vi "CRYGraph Property Window XY.vi"(9 "TabName":string, 10 "Graph VI Ref":refnum<vi>) -> ()   [LabVIEW 2013]
uses:
  <vilib>/Utility/miscctls.llb/LVRowAndColumnTypeDef.ctl
panel:
  in  "Plot PropertyCtrl Ref":refnum<vi>
  in  "Plot Property":string
  in  "SetFormat":bool
  in  "No Data":bool
  out "CursorLineStyle":string
  out "CursorLineWidth":string
  out "CursorPointStyle":string
  out "CursorStyle":string
  out "Scale Style":u8=5
  out "Interpolation":string
  out "PointStyle":string
  out "LineWidth":string
  out "LineStyle":string
  in  "Property Tab":T1(tab)
  in  "Background Color":u32(colorbox)
  in  "Title Name":string
  in  "FormatAxis":u16(ring) items=["X-Axis", "Y-Axis"]
  in  "Notation":i32(listbox)
  in  "PrecisionType":u16(ring) items=["Digitals of precision", "Significant digits"]
  in  "PrecisionDigits":u16
  in  "Hide trailing zeros":bool
  in  "Exponent in multiples of 3":bool
  in  "Use minimum field width":bool
  in  "Field Width":u16
  in  "PadType":u16(ring) items=["Pad with spaces on left", "Pad with spaces on right", "Pad with zeros on left"]
  in  "Ignore timestamp information":bool
  in  "TimeFormat":u16(ring) items=["Custom time format", "System time format", "Time unused"]
  in  "Digits":u16
  in  "DateFormat":u16(ring) items=["Custom date format", "System date format", "Date unused"]
  in  "YMD":u16(slide)
  in  "YearShow":u16(slide)
  in  "AMFM":u16(slide)=1
  in  "HMS":u16(slide)=1
  in  "Point/Fill":u32(colorbox)
  in  "Fill to":i16(ring) items=["none"=-1, "zero"=-2, "-Infinity"=-3, "+Infinity"=-4]
  in  "Items":u16(ring)
  out "Colors":bool
  in  "Line":u32(colorbox)
  in  "LineStyle4":bool
  in  "LineStyle3":bool
  in  "LineStyle2":bool
  in  "LineStyle0":bool
  in  "LineStyle1":bool
  in  "LineWidth5":bool
  in  "LineWidth1":bool
  in  "LineWidth4":bool
  in  "LineWidth3":bool
  in  "LineWidth2":bool
  in  "LineWidth0":bool
  in  "PointStyle16":bool
  in  "PointStyle15":bool
  in  "PointStyle14":bool
  in  "PointStyle13":bool
  in  "PointStyle12":bool
  in  "PointStyle11":bool
  in  "PointStyle10":bool
  in  "PointStyle9":bool
  in  "PointStyle8":bool
  in  "PointStyle7":bool
  in  "PointStyle6":bool
  in  "PointStyle5":bool
  in  "PointStyle4":bool
  in  "PointStyle3":bool
  in  "PointStyle2":bool
  in  "PointStyle1":bool
  in  "PointStyle0":bool
  in  "Interpolation4":bool
  in  "Interpolation5":bool
  in  "Interpolation3":bool
  in  "Interpolation2":bool
  in  "Interpolation1":bool
  in  "Interpolation0":bool
  in  "Show Plot":bool
  in  "GridStyle":u16(ring)=4
  out "Grid Colors":bool
  in  "Minor grid":u32(colorbox)
  in  "Major grid":u32(colorbox)
  in  "Marker text":u32(colorbox)
  in  "Minor tick":u32(colorbox)
  in  "Log":bool
  in  "Show scale":bool
  in  "Show scale label":bool
  in  "Maximum":dbl
  in  "Minimum":dbl
  in  "Autoscale":bool
  in  "Axis Name":string caption="Name"
  in  "Axis":u16(ring)
  in  "Major tick":u32(colorbox)
  out "Scale Style and Colors":bool
  in  "Cursor Tab":enum32{"Page 1"}(tab)
  in  "CursorPointStyle16":bool
  in  "CursorPointStyle15":bool
  in  "CursorPointStyle14":bool
  in  "CursorPointStyle13":bool
  in  "CursorPointStyle12":bool
  in  "CursorPointStyle11":bool
  in  "CursorPointStyle10":bool
  in  "CursorPointStyle9":bool
  in  "CursorPointStyle8":bool
  in  "CursorPointStyle7":bool
  in  "CursorPointStyle6":bool
  in  "CursorPointStyle5":bool
  in  "CursorPointStyle4":bool
  in  "CursorPointStyle3":bool
  in  "CursorPointStyle2":bool
  in  "CursorPointStyle1":bool
  in  "CursorPointStyle0":bool
  in  "CursorLineWidth5":bool
  in  "CursorLineWidth1":bool
  in  "CursorLineWidth4":bool
  in  "CursorLineWidth3":bool
  in  "CursorLineWidth2":bool
  in  "CursorLineWidth0":bool
  in  "CursorLineStyle4":bool
  in  "CursorLineStyle3":bool
  in  "CursorLineStyle2":bool
  in  "CursorLineStyle0":bool
  in  "CursorLineStyle1":bool
  in  "Cursor Items":u16(ring)
  in  "CursorStyle8":bool
  in  "CursorStyle4":bool
  in  "CursorStyle5":bool
  in  "CursorStyle7":bool
  in  "CursorStyle6":bool
  in  "CursorStyle3":bool
  in  "CursorStyle2":bool
  in  "CursorStyle1":bool
  in  "CursorStyle0":bool
  in  "Cursor color":u32(colorbox)
  in  "Linked to plot:":u16(ring)
  in  "Link Cursors":bool
  in  "Show Cursors":bool
  in  "OK":bool
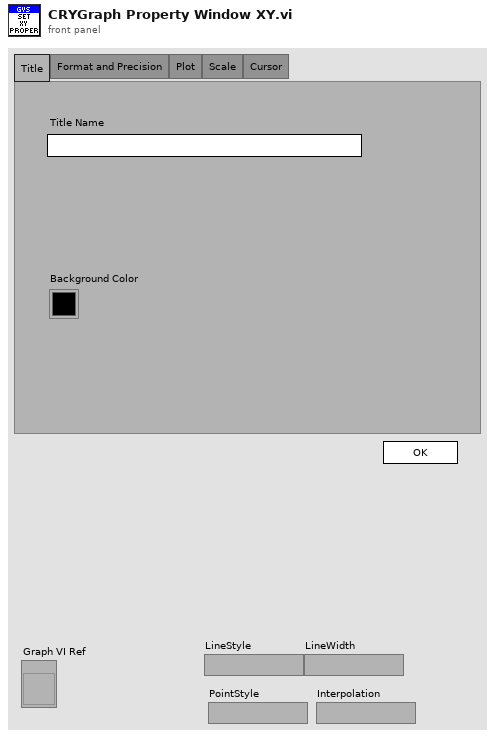
[diagram p1: front panel]
types:
  T1 = enum32{"Title", "Format and Precision", "Plot", "Scale", "Cursor"}
  T2 = enum32{"Page Enabled", "Page Disabled", "Page Disabled & Grayed"}
  T3 = enum8{"Enabled", "Disabled", "Disabled and Grayed Out"}
  T4 = typedef "LVRowAndColumnTypeDef.ctl" = cluster{"Row":i32, "Column":i32}
  T5 = typedef "CRYData Cluster.ctl" = cluster{"Name":string, "Curve":cluster{"x":dbl, "y":dbl, "z":dbl}[], "X data":u16, "Y data":u16, "Z data":u16, "X axis":u16, "Y axis":u16, "Z axis":u16, "X unit":string, "Y unit":string, "Z unit":string, "X dB ref":dbl, "Y dB ref":dbl, "Z dB ref":dbl, "single val":bool, "protected":bool, "display X":bool, "display Y":bool, "display Z":bool, "Test Info":string, "Step No.":i32, "Plot Settings":cluster{"Color":u32, "Interpolation":u8, "Point Style":u8, "Line Style":u8, "Point Color":u32, "Line Width":u8, "Bar Plot Style":u8, "Fill To":i16}, "AutoProtect":bool}
  T6 = cluster{"Notation":i32, "PrecisionType":u16, "PrecisionDigits":u16, "Hide trailing zeros":bool, "Exponent in multiples of 3":bool, "Field Width":u16, "PadType":u16, "Use minimum field width":bool, "TimeFormat":u16, "AMFM":u16, "HMS":u16, "Digits":u16, "DateFormat":u16, "YMD":u16, "YearShow":u16}
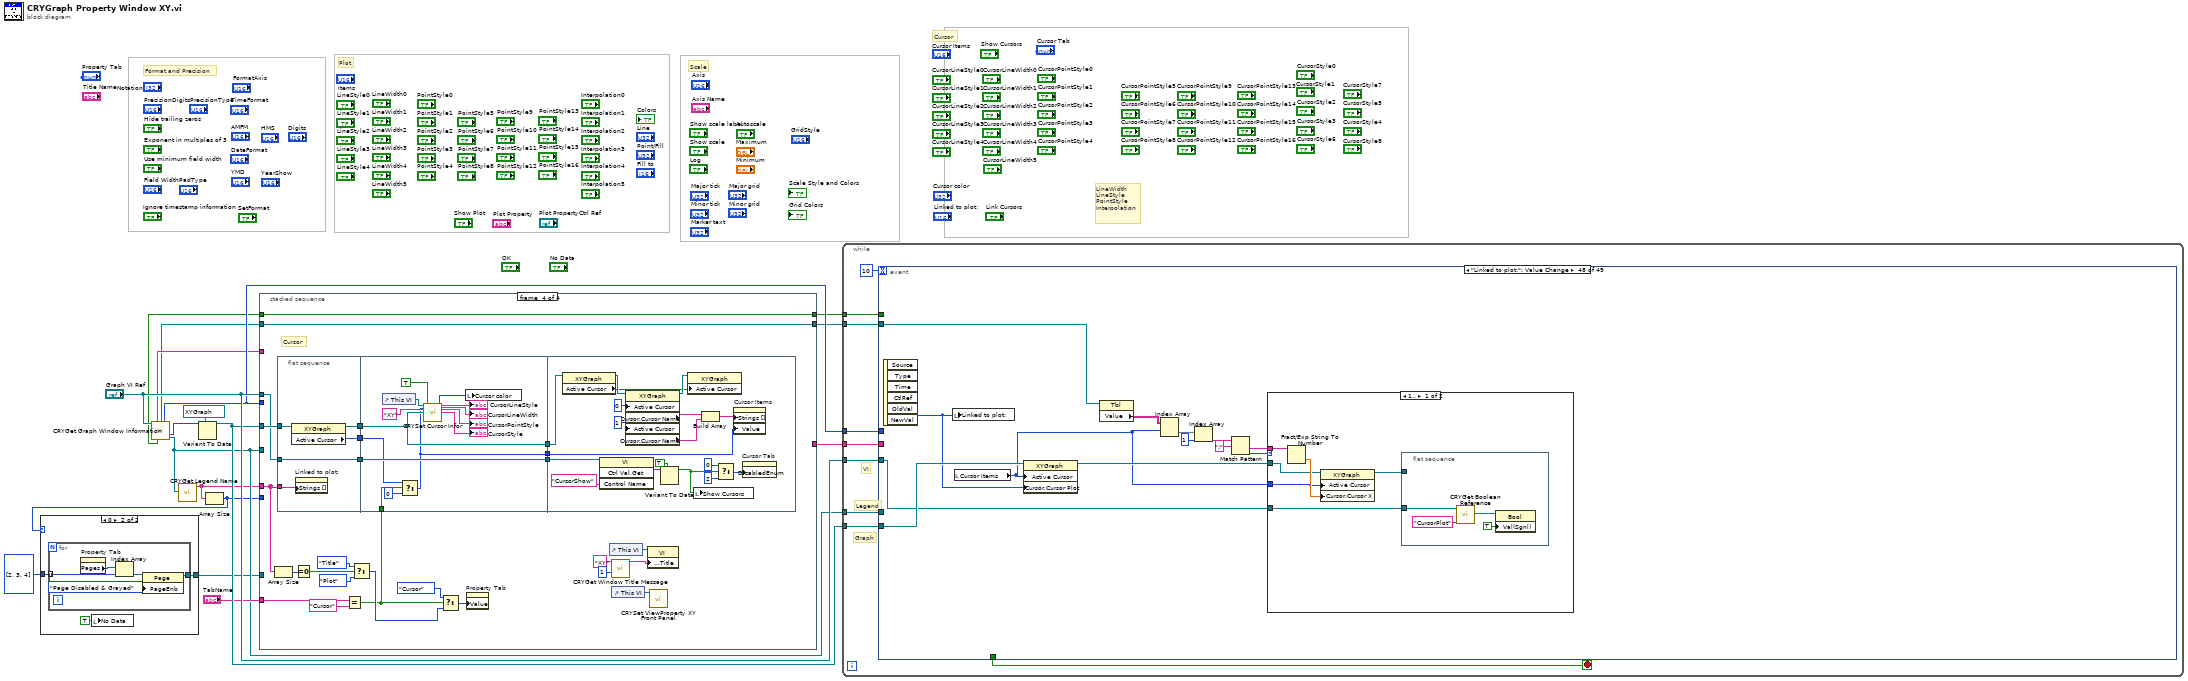
[diagram p0: block diagram]
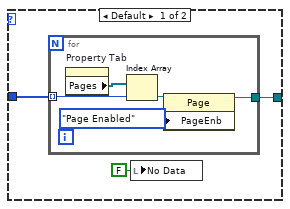
[diagram p2: hidden frame]
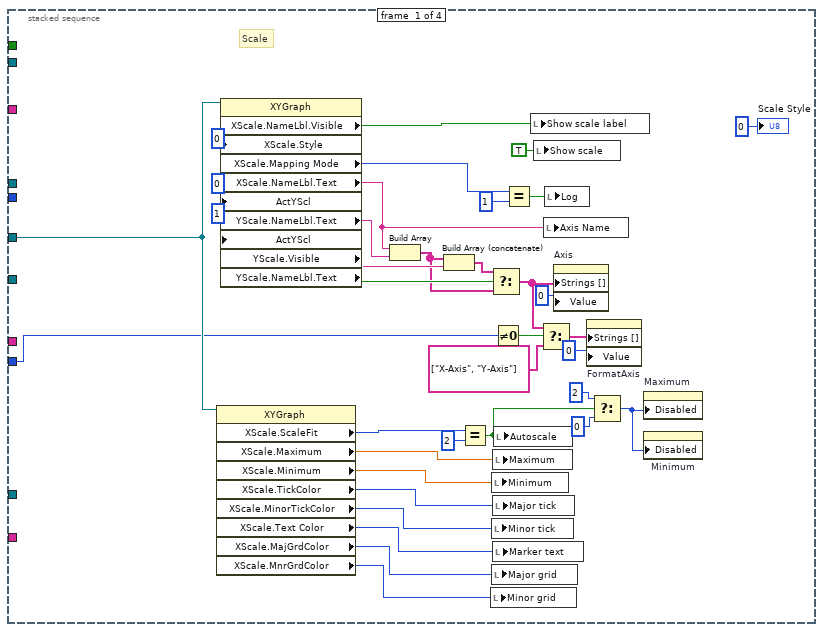
[diagram p3: hidden frame]
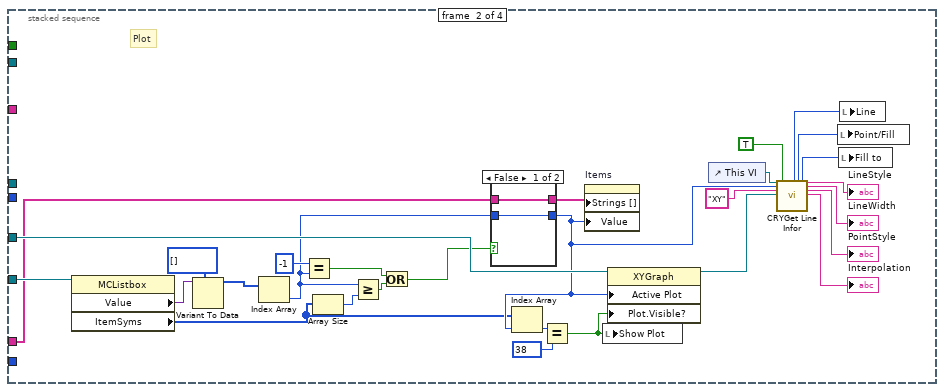
[diagram p4: hidden frame]
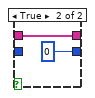
[diagram p5: hidden frame]
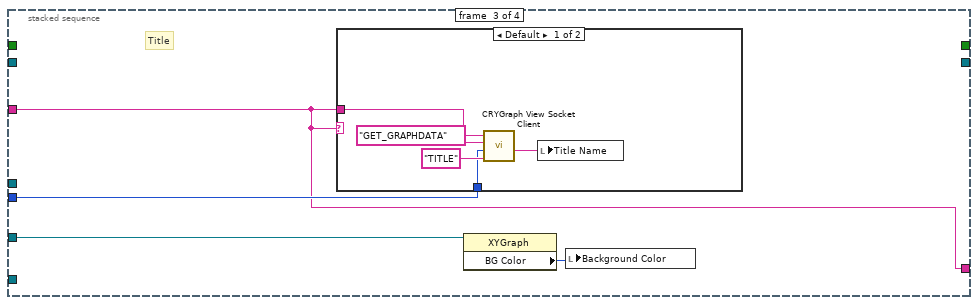
[diagram p6: hidden frame]
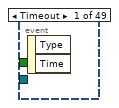
[diagram p8: hidden frame]
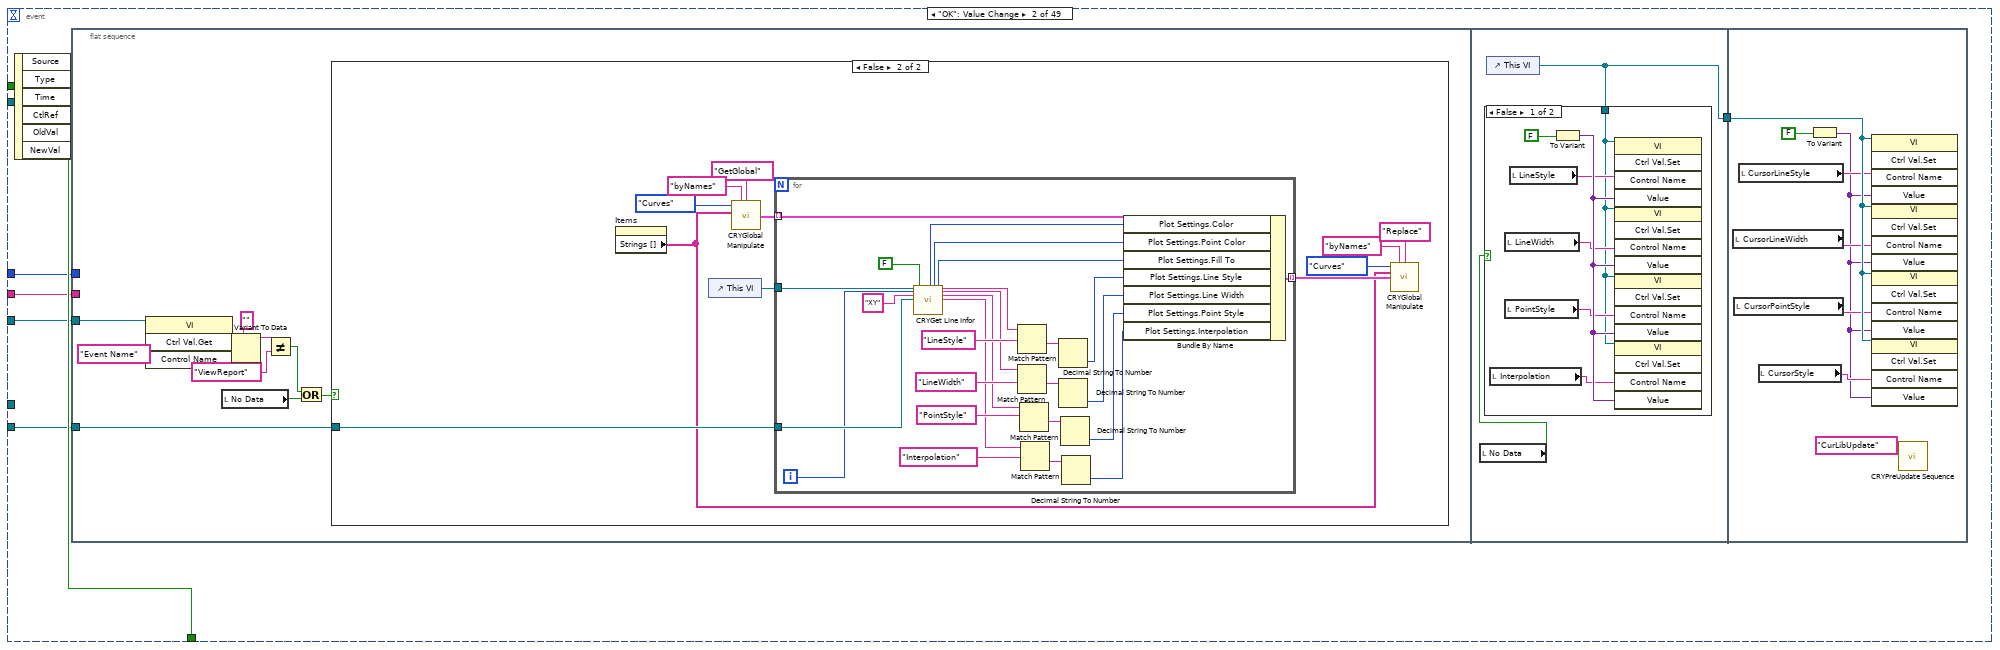
[diagram p9: hidden frame]
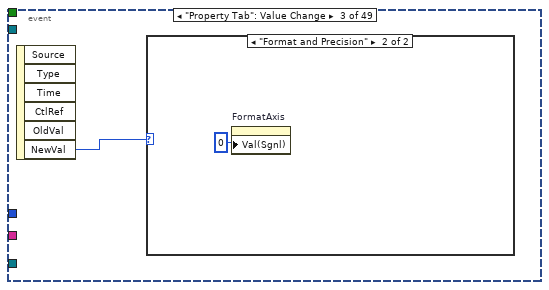
[diagram p12: hidden frame]
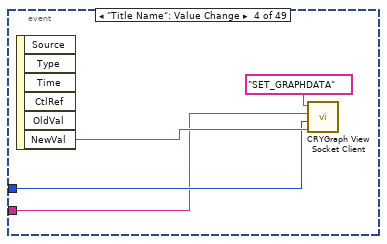
[diagram p14: hidden frame]
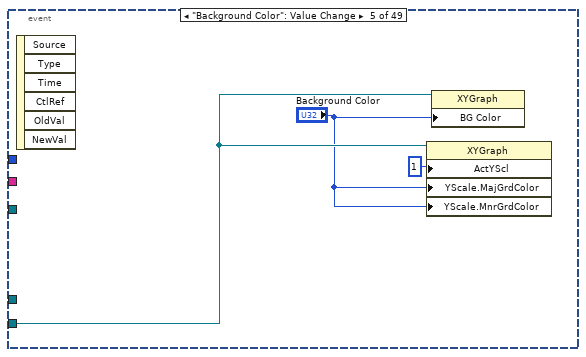
[diagram p15: hidden frame]
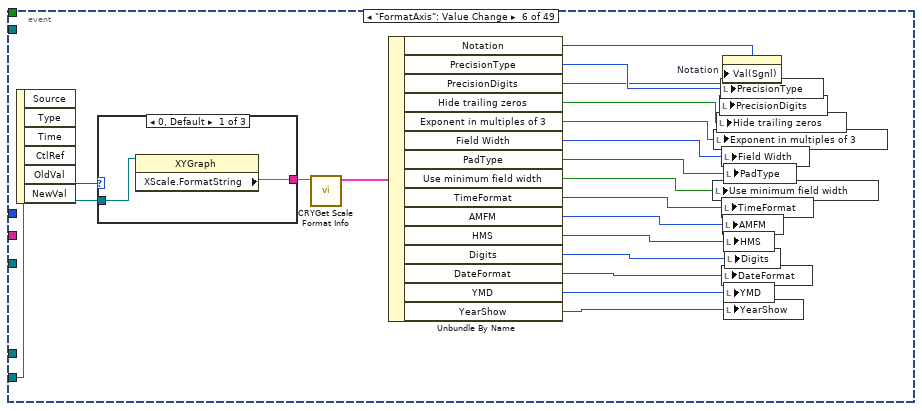
[diagram p16: hidden frame]
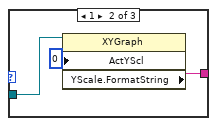
[diagram p17: hidden frame]
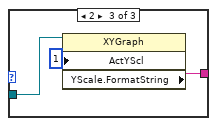
[diagram p18: hidden frame]
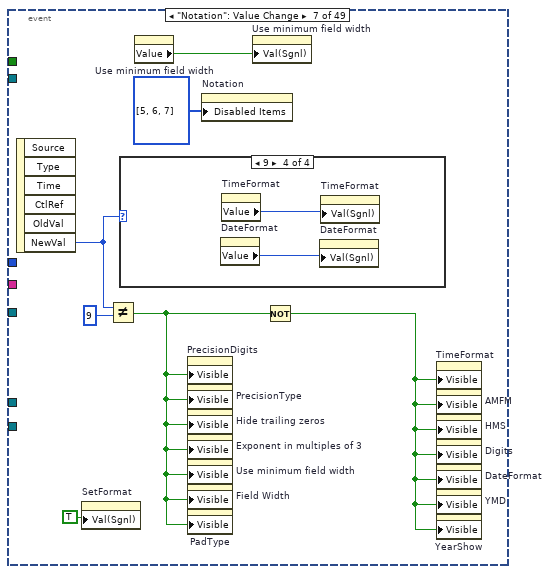
[diagram p19: hidden frame]
diagram:
  # "LineWidth\nLineStyle\nPointStyle\nInterpolation"
  # "Format and Precision"
  # "Cursor"
  # "Scale"
  # "Plot"
  n1 = call "CRYGet Graph Window Information.vi"("pGraph VI In"="Graph VI Ref") -> ("Queue Name Out"=w14:string, "Cursor Ref Out"=w4:refnum<vi>, "Graph Number Out"=w15:i32, "Graph Control Ref Out"=w6:variant, "CursorShow Out"=w2:bool, "Legend Ref Out"=w11:refnum<vi>)  [unwired: 2 in, 7 out]
  n2 = call "CRYGet Legend Name.vi"("MCListbox Refnum"=w11) -> ("Names Out"=w10:string[])  [unwired: 1 in, 9 out]
  n3 = Variant To Data(type=refnum<vi> refnum ("XY Graph"), Variant=w6) -> (data=w16:refnum<vi>)  [unwired: 1 in, 1 out]
  n4 = Array Size(array=w10) -> (size(s)=w9:i32)
  n5 = case shown="0" w9 {
    tunnel: i32[] [2, 3, 4] -> [w19 w27]
    tunnel: [w18 w26] -> w8
    frame Default {
      n6 = for {
        tunnel: w19 -> [w23] mode=indexing
        tunnel: [w21] -> w18
        n7 = property on="Property Tab" class="TabCtl (strict)"() -> ("Pages"=w22:refnum<vi>[])  [unwired: 2 in, 2 out]
        n8 = Index Array(array=w22, index=w23) -> (element=w24:refnum<vi>)
        n9 = property class="Page"(reference=w24, "PageEnb"=T2."Page Enabled" ("Page Enabled State")) -> (reference out=w21:refnum<vi>)  [unwired: 1 in, 1 out]
      }
      n10 = local write "No Data"(FALSE ("No Data")) -> ()
    }
    frame 0 {
      n11 = for {
        tunnel: w27 -> [w30] mode=indexing
        tunnel: [w29] -> w26
        n12 = property on="Property Tab" class="TabCtl (strict)"() -> ("Pages"=w31:refnum<vi>[])  [unwired: 2 in, 2 out]
        n13 = Index Array(array=w31, index=w30) -> (element=w32:refnum<vi>)
        n14 = property class="Page"(reference=w32, "PageEnb"=T2."Page Disabled & Grayed" ("Page Enabled State")) -> (reference out=w29:refnum<vi>)  [unwired: 1 in, 1 out]
      }
      n15 = local write "No Data"(TRUE ("No Data")) -> ()
    }
  }
  n16 = stacked-sequence {
    tunnel: w16 -> [w69 w97 w106 w137]
    tunnel: "Graph VI Ref" -> [_ _ _ w134]
    tunnel: w11 -> [_ w98 _ _]
    tunnel: w15 -> [_ _ w104 _]
    tunnel: w14 -> [_ _ w103 _]
    tunnel: [_ _ w103 _] -> w13
    tunnel: "TabName" -> [_ _ _ w132]
    tunnel: w10 -> [_ w96 _ w126]
    tunnel: w9 -> [w38 _ _ _]
    tunnel: w8 -> [_ _ _ _]
    tunnel: w4 -> [_ _ _ w113]
    tunnel: [_ _ _ w113] -> w3
    tunnel: w2 -> [_ _ _ w112]
    tunnel: [_ _ _ w112] -> w1
    frame #0 {
      # "Scale"
      n17 = property class="XYGraph"(reference=w69) -> ("XScale.ScaleFit"=w56:u8, "XScale.Maximum"=w55:dbl, "XScale.Minimum"=w54:dbl, "XScale.TickColor"=w53:u32, "XScale.MinorTickColor"=w52:u32, "XScale.Text Color"=w51:u32, "XScale.MajGrdColor"=w50:u32, "XScale.MnrGrdColor"=w49:u32)  [unwired: 1 in, 2 out]
      n18 = property class="XYGraph"(reference=w69, "XScale.Style"=u8 0 ("X Scale.Style"), "ActYScl"=0 ("Active Y Scale"), "ActYScl"=1 ("Active Y Scale")) -> ("XScale.NameLbl.Visible"=w67:bool, "XScale.Mapping Mode"=w65:u8, "XScale.NameLbl.Text"=w62:string, "YScale.NameLbl.Text"=w60:string, "YScale.Visible"=w43:bool, "YScale.NameLbl.Text"=w42:string)  [unwired: 1 in, 2 out]
      n19 = Build Array(w62, w60) -> (w40:string[])
      n20 = Build Array (concatenate)(w40, w42) -> (w41:string[])
      n21 = Equal?(x=w56, y=u8 2 ("X Scale.Scale Fit")) -> (x = y?=w45:bool)
      n22 = Select(t=w41, s=w43, f=w40) -> (s? t:f=w36:string[])
      n23 = local write "Minor grid"(w49) -> ()
      n24 = local write "Minimum"(w54) -> ()
      n25 = local write "Minor tick"(w52) -> ()
      n26 = local write "Major grid"(w50) -> ()
      n27 = Not Equal To 0?(x=w38) -> (x != 0?=w37:bool)
      n28 = local write "Maximum"(w55) -> ()
      n29 = local write "Major tick"(w53) -> ()
      n30 = local write "Marker text"(w51) -> ()
      n31 = local write "Autoscale"(w45) -> ()
      n32 = Equal?(x=w65, y=u8 1) -> (x = y?=w66:bool)
      n33 = local write "Show scale label"(w67) -> ()
      n34 = local write "Show scale"(TRUE ("Show scale")) -> ()
      n35 = Select(t=w36, s=w37, f=string[] ["X-Axis", "Y-Axis"]) -> (s? t:f=w34:string[])
      n36 = local write "Axis Name"(w62) -> ()
      n37 = local write "Log"(w66) -> ()
      n38 = property on="Axis" class="Ring (strict)"("Strings []"=w36, "Value"=u16 0) -> ()  [unwired: 2 in, 2 out]
      n39 = property on="FormatAxis" class="Ring (strict)"("Strings []"=w34, "Value"=u16 0) -> ()  [unwired: 2 in, 2 out]
      n40 = Select(t=u8 2 ("X Scale.Scale Fit"), s=w45, f=u8 0 ("X Scale.Scale Fit")) -> (s? t:f=w46:u8)
      n41 = property on="Maximum" class="DigNum (strict)"("Disabled"=w46) -> ()  [unwired: 2 in, 2 out]
      n42 = property on="Minimum" class="DigNum (strict)"("Disabled"=w46) -> ()  [unwired: 2 in, 2 out]
      "Scale Style" <- u8 0 ("X Scale.Scale Fit")
    }
    frame #1 {
      # "Plot"
      n43 = property class="MCListbox"(reference=w98) -> ("Value"=w90:variant, "ItemSyms"=w70:i32[])  [unwired: 1 in, 2 out]
      n44 = Variant To Data(type=i32[] [], Variant=w90) -> (data=w73:i32[])  [unwired: 1 in, 1 out]
      n45 = Index Array(array=w73) -> (element=w71:i32)  [unwired: 1 in]
      n46 = Equal?(x=-1, y=w71) -> (x = y?=w75:bool)
      n47 = Array Size(array=w70) -> (size(s)=w76:i32)
      n48 = Greater Or Equal?(x=w71, y=w76) -> (x >= y?=w74:bool)
      n49 = Or(x=w75, y=w74) -> (x .or. y?=w72:bool)
      n50 = case shown="False" w72 {
        tunnel: w96 -> [w100 w102]
        tunnel: [w100 w102] -> w95
        tunnel: [w99 0 ("Value")] -> w89
        tunnel: w71 -> [w99 _]
        frame False {
        }
        frame True {
        }
      }
      n51 = Index Array(array=w70, index=w89) -> (element=w92:i32)
      n52 = Equal?(x=w92, y=38) -> (x = y?=w91:bool)
      n53 = property on="Items" class="Ring (strict)"("Strings []"=w95, "Value"=w89) -> ()  [unwired: 2 in, 2 out]
      n54 = local write "Show Plot"(w91) -> ()
      n55 = property class="XYGraph"(reference=w97, "Active Plot"=w89, "Plot.Visible?"=w91) -> (reference out=w94:refnum<vi>)  [unwired: 1 in, 1 out]
      n56 = control-ref of="This VI"() -> (w88:refnum<vi>)
      n57 = call "CRYGet Line Infor.vi"("This VI"=w88, "Active Plot Number"=w89, "Graph Type"="XY", "XY Graph Control Ref"=w94, "Property Set?"=TRUE) -> ("Line"=w81:u32, "Point/Fill"=w79:u32, "Fill to"=w80:i16, "LineStyle"=→"LineStyle":string, "LineWidth"=→"LineWidth":string, "PointStyle"=→"PointStyle":string, "Interpolation"=→"Interpolation":string)  [unwired: 16 in]
      n58 = local write "Point/Fill"(w79) -> ()
      n59 = local write "Fill to"(w80) -> ()
      n60 = local write "Line"(w81) -> ()
    }
    frame #2 {
      # "Title"
      n61 = case shown="Default" w103 {
        tunnel: w104 -> [w109 _]
        tunnel: w103 -> [w108 _]
        frame Default {
          n62 = call "CRYGraph View Socket Client.vi"("sOption"="TITLE", "nData"=w109, "sData"=w108, "sAction"="GET_GRAPHDATA") -> ("sData Out"=w107:string)  [unwired: 4 in, 3 out]
          n63 = local write "Title Name"(w107) -> ()
        }
        frame "test DataView" {
        }
      }
      n64 = property class="XYGraph"(reference=w106) -> ("BG Color"=w105:u32)  [unwired: 1 in, 2 out]
      n65 = local write "Background Color"(w105) -> ()
    }
    frame #3 {
      # "Cursor"
      n66 = Array Size(array=w126) -> (size(s)=w133:i32)
      n67 = flat-sequence {
        tunnel: w134 -> [w142]
        tunnel: w137 -> [w140]
        tunnel: [w139] -> w128
        tunnel: [w142] -> w127
        tunnel: w126 -> [w141]
        tunnel: [w138] -> w124
        tunnel: [w156] -> w136
        tunnel: [w147] -> w135
        tunnel: w128 -> [w156]
        tunnel: w127 -> [w147]
        tunnel: w125 -> [w145]
        tunnel: w124 -> [w144]
        tunnel: [w143] -> w123
        tunnel: w136 -> [w160]
        tunnel: w135 -> [w166]
        tunnel: w123 -> [w157]
        frame #0 {
          n68 = property class="XYGraph"(reference=w140) -> (reference out=w139:refnum<vi>, "Active Cursor"=w138:u32)  [unwired: 1 in, 1 out]
          n69 = property on="Linked to plot:" class="Ring (strict)"("Strings []"=w141) -> ()  [unwired: 2 in, 2 out]
        }
        frame #1 {
          n70 = control-ref of="This VI"() -> (w155:refnum<vi>)
          n71 = Select(t=w144, s=w145, f=u32 0 ("Active Cursor")) -> (s? t:f=w143:u32)
          n72 = call "CRYSet Cursor Infor.vi"("This VI"=w155, "Active Cursor"=w143, "Graph Type"="XY", "XY Graph Ref"=w156, "Property Set?"=TRUE) -> ("Cursor Color"=w148:u32, "CursorLineStyle"=→"CursorLineStyle":string, "CursorLineWidth"=→"CursorLineWidth":string, "CursorPointStyle"=→"CursorPointStyle":string, "CursorStyle"=→"CursorStyle":string)  [unwired: 17 in, 1 out]
          n73 = local write "Cursor color"(w148) -> ()
        }
        frame #2 {
          n74 = property class="XYGraph"(reference=w160) -> (reference out=w159:refnum<vi>, "Active Cursor"=w158:u32)  [unwired: 1 in, 1 out]
          n75 = invoke class="VI" method="Ctrl Val.Get"(reference=w166, "Control Name"="CursorShow") -> ("Get Control Value Variant"=w164:variant)  [unwired: 2 in, 3 out]
          n76 = property class="XYGraph"(reference=w159, "Active Cursor"=u32 0, "Active Cursor"=u32 1) -> (reference out=w161:refnum<vi>, "Cursor.Cursor Name"=w169:string, "Cursor.Cursor Name"=w170:string)  [unwired: 1 in, 1 out]
          n77 = Variant To Data(type=TRUE ("Visible"), Variant=w164) -> (data=w162:bool)  [unwired: 1 in, 1 out]
          n78 = property class="XYGraph"(reference=w161, "Active Cursor"=w158) -> ()  [unwired: 1 in, 2 out]
          n79 = local write "Show Cursors"(w162) -> ()
          n80 = Build Array(w169, w170) -> (w171:string[])
          n81 = Select(t=0, s=w162, f=2) -> (s? t:f=w172:i32)
          n82 = property on="Cursor Items" class="Ring (strict)"("Strings []"=w171, "Value"=w157) -> ()  [unwired: 2 in, 2 out]
          n83 = property on="Cursor Tab" class="TabCtl (strict)"("DisabledEnum"=w172) -> ()  [unwired: 2 in, 2 out]
        }
      }
      n84 = Equal To 0?(x=w133) -> (x = 0?=w130:bool)
      n85 = Equal?(x=w132, y="Cursor" ("Graph Type")) -> (x = y?=w125:bool)
      n86 = Select(t=T1."Title" ("Tab Control"), s=w130, f=T1."Plot" ("Tab Control")) -> (s? t:f=w129:T1)
      n87 = Select(t=T1."Cursor" ("Tab Control"), s=w125, f=w129) -> (s? t:f=w119:T1)
      n88 = property on="Property Tab" class="TabCtl (strict)"("Value"=w119) -> ()  [unwired: 2 in, 2 out]
      n89 = control-ref of="This VI"() -> (w115:refnum<vi>)
      n90 = call "CRYGet Window Title Message.vi"("No"=1 ("Error No"), "Kind"="XY") -> ("Multibyte String"=w116:string)  [unwired: 4 in, 5 out]
      n91 = control-ref of="This VI"() -> (w114:refnum<vi>)
      n92 = property class="VI"(reference=w115, "Front Panel.Title"=w116) -> ()  [unwired: 1 in, 2 out]
      n93 = call "CRYSet ViewProperty XY  Front Panel.vi"("Vi Ref"=w114) -> ()  [unwired: 11 in]
    }
  }
  n94 = while {
    tunnel: w16 -> [w182]
    tunnel: "Graph VI Ref" -> [w181]
    tunnel: w11 -> [w179]
    tunnel: w13 -> [w178]
    tunnel: w15 -> [w177]
    tunnel: w3 -> [w176]
    tunnel: w1 -> [w175]
    stop <- w183 stop-if-true
    # "VI"
    # "Legend"
    # "Graph"
    n95 = event shown="[47] \"Linked to plot:\": Value Change" {
      selector: _ -> [_ _ _ _ _ _ _ _ _ _ _ _ _ _ _ _ _ _ _ _ _ _ _ _ _ _ _ _ _ _ _ _ _ _ _ _ _ _ _ _ _ _ _ _ _ _ _ _ _]
      dyn-events: _ -> [_ _ _ _ _ _ _ _ _ _ _ _ _ _ _ _ _ _ _ _ _ _ _ _ _ _ _ _ _ _ _ _ _ _ _ _ _ _ _ _ _ _ _ _ _ _ _ _ _]
      timeout: 10 -> [_ _ _ _ _ _ _ _ _ _ _ _ _ _ _ _ _ _ _ _ _ _ _ _ _ _ _ _ _ _ _ _ _ _ _ _ _ _ _ _ _ _ _ _ _ _ _ _ _]
      tunnel: [_ w189 _ _ _ _ _ _ _ _ _ _ _ _ _ _ _ _ _ _ _ _ _ _ _ _ _ _ _ _ _ _ _ _ _ _ _ _ _ _ _ _ _ _ _ _ _ _ _] -> w183
      tunnel: w182 -> [_ w188 _ _ w261 w281 _ _ _ _ _ _ _ _ _ w347 _ _ _ _ _ w518 w555 w565 w575 w592 w614 w658 w670 w685 w697 w711 w723 w734 w745 w755 w767 w785 w822 w833 _ w850 w870 w891 w912 w933 w958 w978 _]
      tunnel: w181 -> [_ w186 _ _ _ _ _ _ _ _ _ _ _ _ _ _ _ _ _ _ _ _ _ _ _ _ _ _ _ _ _ _ _ _ _ _ _ w784 _ _ w846 _ _ _ _ _ w959 w966 _]
      tunnel: w179 -> [_ _ _ _ _ _ _ _ _ _ _ _ _ _ _ _ _ _ _ _ _ w520 w554 w561 w573 w589 _ _ _ _ _ _ _ _ _ _ _ _ _ _ _ _ _ _ _ _ _ _ _]
      tunnel: w178 -> [_ w184 _ w256 _ _ _ _ _ _ _ _ _ _ _ _ _ _ _ _ _ _ w548 w563 w572 _ _ _ _ _ _ _ _ _ _ _ _ _ _ _ _ _ _ _ _ _ _ _ _]
      tunnel: w177 -> [_ w185 _ w257 _ _ _ _ _ _ _ _ _ _ _ _ _ _ _ _ _ _ _ _ _ _ _ _ _ _ _ _ _ _ _ _ _ _ _ _ _ _ _ _ _ _ _ _ _]
      tunnel: w176 -> [_ _ _ _ _ _ _ _ _ _ _ _ _ _ _ _ _ _ _ _ _ _ _ _ _ _ _ _ _ _ _ _ _ _ _ _ _ _ _ _ _ _ _ _ _ _ _ w976 _]
      tunnel: w175 -> [_ _ _ _ _ _ _ _ _ _ _ _ _ _ _ _ _ _ _ _ _ _ _ _ _ _ _ _ _ _ _ _ _ _ _ _ _ _ _ _ _ _ _ _ _ _ _ _ _]
      event Timeout {
        n96 = event-data() -> ()  [unwired: 3 out]
      }
      event "OK": Value Change {
        n97 = event-data() -> ("NewVal"=w189:bool)  [unwired: 6 out]
        n98 = flat-sequence {
          tunnel: w188 -> [w199]
          tunnel: w186 -> [w190]
          tunnel: w185 -> [_]
          tunnel: w184 -> [_]
          tunnel: [w238] -> w187
          tunnel: w187 -> [w253]
          frame #0 {
            n99 = invoke class="VI" method="Ctrl Val.Get"(reference=w190, "Control Name"="Event Name") -> ("Get Control Value Variant"=w193:variant)  [unwired: 2 in, 3 out]
            n100 = local read "No Data"() -> (w198:bool)
            n101 = Variant To Data(type="" ("Control Name"), Variant=w193) -> (data=w195:string)  [unwired: 1 in, 1 out]
            n102 = Not Equal?(x=w195, y="ViewReport" ("regular expression")) -> (x != y?=w191:bool)
            n103 = Or(x=w191, y=w198) -> (x .or. y?=w197:bool)
            n104 = case shown="False" w197 {
              tunnel: w199 -> [_ w209]
              frame True {
              }
              frame False {
                n105 = property on="Items" class="Ring (strict)"() -> ("Strings []"=w201:string[])  [unwired: 2 in, 2 out]
                n106 = control-ref of="This VI"() -> (w210:refnum<vi>)
                n107 = call "CRYGlobal Manipulate.vi"("Type"=enum16{"Curves", "Values", "Results", "WFM"}."Curves" ("Type In"), "sOption"="byNames", "sAction"="GetGlobal", "sData"=w201) -> ("Curves Out"=w206:T5[])  [unwired: 5 in, 6 out]
                n108 = for {
                  tunnel: w210 -> [w235]
                  tunnel: w209 -> [w234]
                  tunnel: w206 -> [w212] mode=indexing
                  tunnel: [w211] -> w205 mode=indexing
                  i -> [w218]
                  n109 = call "CRYGet Line Infor.vi"("This VI"=w235, "Active Plot Number"=w218, "Graph Type"="XY", "XY Graph Control Ref"=w234, "Property Set?"=FALSE) -> ("Line"=w213:u32, "Point/Fill"=w214:u32, "Fill to"=w215:i16, "LineStyle"=w225:string, "LineWidth"=w221:string, "PointStyle"=w220:string, "Interpolation"=w219:string)  [unwired: 16 in]
                  n110 = Match Pattern(string=w225, regular expression="LineStyle") -> (after substring=w231:string)  [unwired: 4 out]
                  n111 = Match Pattern(string=w221, regular expression="LineWidth") -> (after substring=w232:string)  [unwired: 4 out]
                  n112 = Match Pattern(string=w220, regular expression="PointStyle") -> (after substring=w230:string)  [unwired: 4 out]
                  n113 = Match Pattern(string=w219, regular expression="Interpolation") -> (after substring=w227:string)  [unwired: 4 out]
                  n114 = Decimal String To Number(string=w231) -> (number=w224:i32)  [unwired: 3 out]
                  n115 = Decimal String To Number(string=w232) -> (number=w223:i32)  [unwired: 3 out]
                  n116 = Decimal String To Number(string=w230) -> (number=w222:i32)  [unwired: 3 out]
                  n117 = Decimal String To Number(string=w227) -> (number=w217:i32)  [unwired: 3 out]
                  n118 = Bundle By Name(cluster=w212, "Plot Settings.Color"=w213, "Plot Settings.Point Color"=w214, "Plot Settings.Fill To"=w215, "Plot Settings.Line Style"=w224, "Plot Settings.Line Width"=w223, "Plot Settings.Point Style"=w222, "Plot Settings.Interpolation"=w217) -> (w211:T5)
                }
                n119 = call "CRYGlobal Manipulate.vi"("Type"=enum16{"Curves", "Values", "Results", "WFM"}."Curves", "sOption"="byNames", "sAction"="Replace", "sData"=w201, "Curves"=w205) -> ()  [unwired: 4 in, 7 out]
              }
            }
          }
          frame #1 {
            n120 = local read "No Data"() -> (w237:bool)
            n121 = control-ref of="This VI"() -> (w238:refnum<vi>)
            n122 = case shown="False" w237 {
              tunnel: w238 -> [w239 _]
              frame False {
                n123 = local read "Interpolation"() -> (w240:string)
                n124 = local read "LineWidth"() -> (w242:string)
                n125 = local read "PointStyle"() -> (w241:string)
                n126 = local read "LineStyle"() -> (w243:string)
                n127 = To Variant(anything=FALSE) -> (Variant=w245:variant)
                n128 = invoke class="VI" method="Ctrl Val.Set"(reference=w239, "Control Name"=w243, "Value"=w245) -> ()  [unwired: 2 in, 5 out]
                n129 = invoke class="VI" method="Ctrl Val.Set"(reference=w239, "Control Name"=w242, "Value"=w245) -> ()  [unwired: 2 in, 5 out]
                n130 = invoke class="VI" method="Ctrl Val.Set"(reference=w239, "Control Name"=w241, "Value"=w245) -> ()  [unwired: 2 in, 5 out]
                n131 = invoke class="VI" method="Ctrl Val.Set"(reference=w239, "Control Name"=w240, "Value"=w245) -> ()  [unwired: 2 in, 5 out]
              }
              frame True {
              }
            }
          }
          frame #2 {
            n132 = local read "CursorLineWidth"() -> (w250:string)
            n133 = local read "CursorPointStyle"() -> (w251:string)
            n134 = local read "CursorLineStyle"() -> (w249:string)
            n135 = local read "CursorStyle"() -> (w252:string)
            n136 = To Variant(anything=FALSE) -> (Variant=w247:variant)
            n137 = invoke class="VI" method="Ctrl Val.Set"(reference=w253, "Control Name"=w249, "Value"=w247) -> ()  [unwired: 2 in, 5 out]
            n138 = invoke class="VI" method="Ctrl Val.Set"(reference=w253, "Control Name"=w250, "Value"=w247) -> ()  [unwired: 2 in, 5 out]
            n139 = invoke class="VI" method="Ctrl Val.Set"(reference=w253, "Control Name"=w251, "Value"=w247) -> ()  [unwired: 2 in, 5 out]
            n140 = invoke class="VI" method="Ctrl Val.Set"(reference=w253, "Control Name"=w252, "Value"=w247) -> ()  [unwired: 2 in, 5 out]
            n141 = call "CRYPreUpdate Sequence.vi"("EventName"="CurLibUpdate") -> ()  [unwired: 15 in]
          }
        }
      }
      event "Property Tab": Value Change {
        n142 = event-data() -> ("NewVal"=w254:T1)  [unwired: 6 out]
        n143 = case shown="\"Format and Precision\"" w254 {
          frame "Title", Default {
          }
          frame "Format and Precision" {
            n144 = property on="FormatAxis" class="Ring (strict)"("Val(Sgnl)"=u16 0 ("Value (Signaling)")) -> ()  [unwired: 2 in, 2 out]
          }
        }
      }
      event "Title Name": Value Change {
        n145 = event-data() -> ("NewVal"=w258:string)  [unwired: 6 out]
        n146 = call "CRYGraph View Socket Client.vi"("sOption"=w258, "nData"=w257, "sData"=w256, "sAction"="SET_GRAPHDATA") -> ()  [unwired: 4 in, 4 out]
      }
      event "Background Color": Value Change {
        n147 = event-data() -> ()  [unwired: 7 out]
        n148 = property on="Property Node" class="XYGraph"(reference=w261, "ActYScl"=1 ("Active Y Scale"), "YScale.MajGrdColor"="Background Color", "YScale.MnrGrdColor"="Background Color") -> ()  [unwired: 1 in, 2 out]
        n149 = property class="XYGraph"(reference=w261, "BG Color"="Background Color") -> ()  [unwired: 1 in, 2 out]
      }
      event "FormatAxis": Value Change {
        n150 = event-data() -> ("NewVal"=w280:u16)  [unwired: 6 out]
        n151 = case shown="0, Default" w280 {
          tunnel: w281 -> [w283 w286 w289]
          tunnel: [w282 w284 w287] -> w279
          frame 0, Default {
            n152 = property class="XYGraph"(reference=w283) -> ("XScale.FormatString"=w282:string)  [unwired: 1 in, 2 out]
          }
          frame 1 {
            n153 = property class="XYGraph"(reference=w286, "ActYScl"=0 ("Active Y Scale")) -> ("YScale.FormatString"=w284:string)  [unwired: 1 in, 2 out]
          }
          frame 2 {
            n154 = property class="XYGraph"(reference=w289, "ActYScl"=1 ("Active Y Scale")) -> ("YScale.FormatString"=w287:string)  [unwired: 1 in, 2 out]
          }
        }
        n155 = call "CRYGet Scale Format Info.vi"("FormatString"=w279) -> ("ScaleFormat"=w278:T6)  [unwired: 10 in]
        n156 = Unbundle By Name(w278) -> ("Notation"=w277:i32, "PrecisionType"=w264:u16, "PrecisionDigits"=w263:u16, "Hide trailing zeros"=w276:bool, "Exponent in multiples of 3"=w275:bool, "Field Width"=w274:u16, "PadType"=w273:u16, "Use minimum field width"=w272:bool, "TimeFormat"=w271:u16, "AMFM"=w270:u16, "HMS"=w269:u16, "Digits"=w268:u16, "DateFormat"=w267:u16, "YMD"=w266:u16, "YearShow"=w265:u16)
        n157 = local write "Use minimum field width"(w272) -> ()
        n158 = local write "Exponent in multiples of 3"(w275) -> ()
        n159 = local write "Hide trailing zeros"(w276) -> ()
        n160 = local write "PrecisionDigits"(w263) -> ()
        n161 = local write "PrecisionType"(w264) -> ()
        n162 = local write "Field Width"(w274) -> ()
        n163 = local write "TimeFormat"(w271) -> ()
        n164 = local write "DateFormat"(w267) -> ()
        n165 = property on="Notation" class="LstBox (strict)"("Val(Sgnl)"=w277) -> ()  [unwired: 2 in, 2 out]
        n166 = local write "AMFM"(w270) -> ()
        n167 = local write "PadType"(w273) -> ()
        n168 = local write "HMS"(w269) -> ()
        n169 = local write "YMD"(w266) -> ()
        n170 = local write "YearShow"(w265) -> ()
        n171 = local write "Digits"(w268) -> ()
      }
      event "Notation": Value Change {
        n172 = event-data() -> ("NewVal"=w293:i32)  [unwired: 6 out]
        n173 = property on="SetFormat" class="Bool (strict)"("Val(Sgnl)"=TRUE ("Value (Signaling)")) -> ()  [unwired: 2 in, 2 out]
        n174 = Not Equal?(x=w293, y=9) -> (x != y?=w291:bool)
        n175 = case shown="9" w293 {
          frame Default {
          }
          frame 0, 3 {
            n176 = property on="Exponent in multiples of 3" class="Bool (strict)"("DisabledEnum"=T3."Enabled" ("Disabled")) -> ()  [unwired: 2 in, 2 out]
          }
          frame 1, 2 {
            n177 = property on="Exponent in multiples of 3" class="Bool (strict)"("DisabledEnum"=T3."Disabled and Grayed Out" ("Disabled")) -> ()  [unwired: 2 in, 2 out]
          }
          frame 9 {
            n178 = property on="DateFormat" class="Ring (strict)"() -> ("Value"=w299:u16)  [unwired: 2 in, 2 out]
            n179 = property on="TimeFormat" class="Ring (strict)"() -> ("Value"=w300:u16)  [unwired: 2 in, 2 out]
            n180 = property on="DateFormat" class="Ring (strict)"("Val(Sgnl)"=w299) -> ()  [unwired: 2 in, 2 out]
            n181 = property on="TimeFormat" class="Ring (strict)"("Val(Sgnl)"=w300) -> ()  [unwired: 2 in, 2 out]
          }
        }
        n182 = property on="Use minimum field width" class="Bool (strict)"() -> ("Value"=w296:bool)  [unwired: 2 in, 2 out]
        n183 = property on="PrecisionDigits" class="DigNum (strict)"("Visible"=w291) -> ()  [unwired: 2 in, 2 out]
        n184 = property on="PrecisionType" class="Ring (strict)"("Visible"=w291) -> ()  [unwired: 2 in, 2 out]
        n185 = property on="Hide trailing zeros" class="Bool (strict)"("Visible"=w291) -> ()  [unwired: 2 in, 2 out]
        n186 = property on="Exponent in multiples of 3" class="Bool (strict)"("Visible"=w291) -> ()  [unwired: 2 in, 2 out]
        n187 = property on="Use minimum field width" class="Bool (strict)"("Visible"=w291) -> ()  [unwired: 2 in, 2 out]
        n188 = property on="Field Width" class="DigNum (strict)"("Visible"=w291) -> ()  [unwired: 2 in, 2 out]
        n189 = property on="PadType" class="Ring (strict)"("Visible"=w291) -> ()  [unwired: 2 in, 2 out]
        n190 = property on="Notation" class="LstBox (strict)"("Disabled Items"=i32[] [5, 6, 7]) -> ()  [unwired: 2 in, 2 out]
        n191 = property on="Use minimum field width" class="Bool (strict)"("Val(Sgnl)"=w296) -> ()  [unwired: 2 in, 2 out]
        n192 = Not(x=w291) -> (.not. x?=w292:bool)
        n193 = property on="TimeFormat" class="Ring (strict)"("Visible"=w292) -> ()  [unwired: 2 in, 2 out]
        n194 = property on="AMFM" class="Slide (strict)"("Visible"=w292) -> ()  [unwired: 2 in, 2 out]
        n195 = property on="HMS" class="Slide (strict)"("Visible"=w292) -> ()  [unwired: 2 in, 2 out]
        n196 = property on="Digits" class="DigNum (strict)"("Visible"=w292) -> ()  [unwired: 2 in, 2 out]
        n197 = property on="DateFormat" class="Ring (strict)"("Visible"=w292) -> ()  [unwired: 2 in, 2 out]
        n198 = property on="YMD" class="Slide (strict)"("Visible"=w292) -> ()  [unwired: 2 in, 2 out]
        n199 = property on="YearShow" class="Slide (strict)"("Visible"=w292) -> ()  [unwired: 2 in, 2 out]
      }
      event "PrecisionType", "PrecisionDigits", "Hide trailing zeros", "Exponent in multiples of 3", "PadType": Value Change {
        n200 = event-data() -> ()  [unwired: 7 out]
        n201 = property on="SetFormat" class="Bool (strict)"("Val(Sgnl)"=TRUE ("Value (Signaling)")) -> ()  [unwired: 2 in, 2 out]
      }
      event "Use minimum field width": Value Change {
        n202 = event-data() -> ("NewVal"=w307:bool)  [unwired: 6 out]
        n203 = property on="Field Width" class="DigNum (strict)"() -> ("Value"=w306:u16)  [unwired: 2 in, 2 out]
        n204 = Equal To 0?(x=w306) -> (x = 0?=w311:bool)
        n205 = Select(t=u16 1 ("Field Width"), s=w311, f=w306) -> (s? t:f=w313:u16)
        n206 = Select(t=T3."Enabled" ("Disabled"), s=w307, f=T3."Disabled and Grayed Out") -> (s? t:f=w302:T3)
        n207 = Select(t=w313, s=w307, f=u16 0 ("Field Width")) -> (s? t:f=w305:u16)
        n208 = property on="Field Width" class="DigNum (strict)"("Value"=w305) -> (error out=w303:errorcluster)  [unwired: 2 in, 1 out]
        n209 = property on="Field Width" class="DigNum (strict)"("DisabledEnum"=w302) -> ()  [unwired: 2 in, 2 out]
        n210 = property on="PadType" class="Ring (strict)"("DisabledEnum"=w302) -> ()  [unwired: 2 in, 2 out]
        n211 = property on="SetFormat" class="Bool (strict)"(error in=w303, "Val(Sgnl)"=TRUE ("Value (Signaling)")) -> ()  [unwired: 1 in, 2 out]
      }
      event "Field Width": Value Change {
        n212 = event-data() -> ("NewVal"=w317:u16)  [unwired: 6 out]
        n213 = property on="SetFormat" class="Bool (strict)"("Val(Sgnl)"=TRUE ("Value (Signaling)")) -> ()  [unwired: 2 in, 2 out]
        n214 = Equal To 0?(x=w317) -> (x = 0?=w320:bool)
        n215 = Select(t=T3."Disabled and Grayed Out" ("Disabled"), s=w320, f=T3."Enabled" ("Disabled")) -> (s? t:f=w315:T3)
        n216 = Select(t=FALSE ("x = 0?"), s=w320, f=TRUE ("x = 0?")) -> (s? t:f=w314:bool)
        n217 = property on="Field Width" class="DigNum (strict)"("DisabledEnum"=w315) -> ()  [unwired: 2 in, 2 out]
        n218 = property on="PadType" class="Ring (strict)"("DisabledEnum"=w315) -> ()  [unwired: 2 in, 2 out]
        n219 = property on="Use minimum field width" class="Bool (strict)"("Value"=w314) -> ()  [unwired: 2 in, 2 out]
      }
      event "TimeFormat": Value Change {
        n220 = event-data() -> ("NewVal"=w326:u16)  [unwired: 6 out]
        n221 = case shown="0, Default" w326 {
          tunnel: [T3."Enabled" ("Disabled") T3."Disabled and Grayed Out" ("Disabled") T3."Disabled and Grayed Out" ("Disabled")] -> w324
          tunnel: [T3."Enabled" ("Disabled") T3."Enabled" ("Disabled") T3."Disabled and Grayed Out" ("Disabled")] -> w323
          frame 0, Default {
            n222 = property on="HMS" class="Slide (strict)"() -> ("Value"=w327:u16)  [unwired: 2 in, 2 out]
            n223 = property on="HMS" class="Slide (strict)"("Val(Sgnl)"=w327) -> ()  [unwired: 2 in, 2 out]
          }
          frame 1 {
          }
          frame 2 {
          }
        }
        n224 = property on="SetFormat" class="Bool (strict)"("Val(Sgnl)"=TRUE ("Value (Signaling)")) -> ()  [unwired: 2 in, 2 out]
        n225 = property on="AMFM" class="Slide (strict)"("DisabledEnum"=w324) -> ()  [unwired: 2 in, 2 out]
        n226 = property on="HMS" class="Slide (strict)"("DisabledEnum"=w324) -> ()  [unwired: 2 in, 2 out]
        n227 = property on="Digits" class="DigNum (strict)"("DisabledEnum"=w323) -> ()  [unwired: 2 in, 2 out]
      }
      event "AMFM", "Digits", "YMD", "YearShow": Value Change {
        n228 = event-data() -> ()  [unwired: 7 out]
        n229 = property on="SetFormat" class="Bool (strict)"("Val(Sgnl)"=TRUE ("Value (Signaling)")) -> ()  [unwired: 2 in, 2 out]
      }
      event "HMS": Value Change {
        n230 = event-data() -> ("NewVal"=w337:u16)  [unwired: 6 out]
        n231 = property on="SetFormat" class="Bool (strict)"("Val(Sgnl)"=TRUE ("Value (Signaling)")) -> ()  [unwired: 2 in, 2 out]
        n232 = Equal To 0?(x=w337) -> (x = 0?=w338:bool)
        n233 = Select(t=T3."Disabled and Grayed Out" ("Disabled"), s=w338, f=T3."Enabled" ("Disabled")) -> (s? t:f=w335:T3)
        n234 = property on="Digits" class="DigNum (strict)"("DisabledEnum"=w335) -> ()  [unwired: 2 in, 2 out]
      }
      event "DateFormat": Value Change {
        n235 = event-data() -> ("NewVal"=w343:u16)  [unwired: 6 out]
        n236 = case shown="0, Default" w343 {
          tunnel: [T3."Enabled" ("Disabled") T3."Disabled and Grayed Out" ("Disabled")] -> w341
          frame 0, Default {
          }
          frame 1, 2 {
          }
        }
        n237 = property on="SetFormat" class="Bool (strict)"("Val(Sgnl)"=TRUE ("Value (Signaling)")) -> ()  [unwired: 2 in, 2 out]
        n238 = property on="YMD" class="Slide (strict)"("DisabledEnum"=w341) -> ()  [unwired: 2 in, 2 out]
        n239 = property on="YearShow" class="Slide (strict)"("DisabledEnum"=w341) -> ()  [unwired: 2 in, 2 out]
      }
      event "Ignore timestamp information": Value Change {
        n240 = event-data() -> ()  [unwired: 7 out]
        n241 = property on="SetFormat" class="Bool (strict)"("Val(Sgnl)"=TRUE ("Value (Signaling)")) -> ()  [unwired: 2 in, 2 out]
      }
      event "SetFormat": Value Change {
        n242 = event-data() -> ()  [unwired: 7 out]
        n243 = local read "Notation"() -> (w350:i32)
        n244 = case shown="0..3, 5..7, Default" w350 {
          tunnel: w350 -> [w368 _]
          tunnel: [w367 w407] -> w349
          frame 0..3, 5..7, Default {
            # "%[$][-][+][#][^][0][Width][.Precision || _SignificantDigits][{Unit}][<Embedded information>]Conversion"
            n245 = local read "Exponent in multiples of 3"() -> (w364:bool)
            n246 = local read "Use minimum field width"() -> (w361:bool)
            n247 = local read "Hide trailing zeros"() -> (w365:bool)
            n248 = local read "PrecisionDigits"() -> (w359:u16)
            n249 = local read "PrecisionType"() -> (w360:u16)
            n250 = local read "Field Width"() -> (w362:u16)
            n251 = local read "PadType"() -> (w363:u16)
            n252 = Select(t="#" ("format string"), s=w365, f="" ("format string")) -> (s? t:f=w377:string)
            n253 = Select(t="^" ("format string"), s=w364, f="" ("format string")) -> (s? t:f=w380:string)
            n254 = case shown="True" w361 {
              tunnel: w363 -> [_ w394]
              tunnel: w362 -> [_ w389]
              tunnel: [w386 w393] -> w382
              tunnel: [w386 w387] -> w383
              tunnel: [w386 w392] -> w381
              frame False {
                w386 = ""
              }
              frame True {
                n255 = Not Equal To 0?(x=w389) -> (x != 0?=w390:bool)
                n256 = case shown="2" w394 {
                  tunnel: [w395 "" ("format string") "0" ("format string")] -> w393
                  tunnel: [w395 "-" ("format string") "" ("format string")] -> w392
                  frame 0, Default {
                    w395 = "" ("format string")
                  }
                  frame 1 {
                  }
                  frame 2 {
                  }
                }
                n257 = Number To Decimal String(number=w389) -> (decimal integer string=w388:string)  [unwired: 1 in]
                n258 = Select(t=w388, s=w390, f="") -> (s? t:f=w387:string)
              }
            }
            n259 = Number To Decimal String(number=w359) -> (decimal integer string=w366:string)  [unwired: 1 in]
            n260 = Equal?(x=w360, y=u16 0) -> (x = y?=w374:bool)
            n261 = Index Array(array=string[] ["f", "e", "g", "p", "", "x", "o", "b", "", "T"], index=w368) -> (element=w385:string)
            n262 = Select(t="." ("format string"), s=w374, f="_" ("format string")) -> (s? t:f=w384:string)
            n263 = Concatenate Strings("%" ("string"), w381, w377, w380, w382, w383, w384, w366, w385) -> (w367:string)
          }
          frame 9 {
            n264 = local read "DateFormat"() -> (w402:u16)
            n265 = local read "TimeFormat"() -> (w406:u16)
            n266 = local read "YearShow"() -> (w400:u16)
            n267 = local read "AMFM"() -> (w405:u16)
            n268 = local read "Digits"() -> (w403:u16)
            n269 = local read "HMS"() -> (w404:u16)
            n270 = local read "YMD"() -> (w401:u16)
            n271 = Equal?(x=w402, y=u16 2) -> (x = y?=w422:bool)
            n272 = Equal?(x=w406, y=u16 2) -> (x = y?=w421:bool)
            n273 = case shown="0, Default" w406 {
              tunnel: w405 -> [w481 _ _]
              tunnel: w404 -> [w479 _ _]
              tunnel: w403 -> [w465 w483 _]
              tunnel: [w468 w482 w485] -> w408
              tunnel: w402 -> [_ _ w490]
              frame 0, Default {
                # "Custom Format"
                n274 = Equal To 0?(x=w481) -> (x = 0?=w472:bool)
                n275 = Not Equal To 0?(x=w465) -> (x != 0?=w467:bool)
                n276 = Equal To 0?(x=w479) -> (x = 0?=w476:bool)
                n277 = Format Into String(format string=":%%S%%%du", w465) -> (resulting string=w464:string)  [unwired: 2 in, 1 out]
                n278 = Select(t="%I:%M" ("format string"), s=w472, f="%H:%M" ("format string")) -> (s? t:f=w477:string)
                n279 = Select(t=w464, s=w467, f=":%S" ("format string")) -> (s? t:f=w463:string)
                n280 = Select(t="", s=w476, f=w463) -> (s? t:f=w473:string)
                n281 = Select(t=" %p", s=w472, f="" ("t")) -> (s? t:f=w469:string)
                n282 = Concatenate Strings(w477, w473, w469) -> (w468:string)
              }
              frame 1 {
                # "System Format"
                n283 = Format Into String(format string="%%.%dX", w483) -> (resulting string=w482:string)  [unwired: 2 in, 1 out]
              }
              frame 2 {
                # "No Used"
                n284 = Equal?(x=w490, y=u16 2) -> (x = y?=w488:bool)
                n285 = Select(t="%.3X" ("format string"), s=w488, f="") -> (s? t:f=w485:string)
              }
            }
            n286 = case shown="0, Default" w402 {
              tunnel: w401 -> [w431 _ _]
              tunnel: w400 -> [w430 _ _]
              tunnel: [w428 "%x" ("format string") w457] -> w409
              tunnel: w406 -> [_ _ w458]
              frame 0, Default {
                # "Custom Format"
                n287 = case shown="2" w430 {
                  tunnel: ["" ("format string") "%y" ("format string") "%Y" ("format string")] -> w429
                  frame 0, Default {
                  }
                  frame 1 {
                  }
                  frame 2 {
                  }
                }
                n288 = case shown="2" w431 {
                  tunnel: w429 -> [w436 w443 w451]
                  tunnel: [w440 w447 w455] -> w428
                  frame 0, Default {
                    n289 = Empty String/Path?(string/path=w436) -> (empty?=w439:bool)
                    n290 = Concatenate Strings("/" ("string"), w436) -> (w437:string)
                    n291 = Select(t=w436, s=w439, f=w437) -> (s? t:f=w438:string)
                    n292 = Concatenate Strings("%m/%d" ("format string"), w438) -> (w440:string)
                  }
                  frame 1 {
                    n293 = Empty String/Path?(string/path=w443) -> (empty?=w446:bool)
                    n294 = Concatenate Strings("/" ("string"), w443) -> (w444:string)
                    n295 = Select(t=w443, s=w446, f=w444) -> (s? t:f=w445:string)
                    n296 = Concatenate Strings("%d/%m" ("format string"), w445) -> (w447:string)
                  }
                  frame 2 {
                    n297 = Empty String/Path?(string/path=w451) -> (empty?=w454:bool)
                    n298 = Concatenate Strings(w451, "/" ("string")) -> (w453:string)
                    n299 = Select(t=w451, s=w454, f=w453) -> (s? t:f=w450:string)
                    n300 = Concatenate Strings(w450, "%m/%d" ("format string")) -> (w455:string)
                  }
                }
              }
              frame 1 {
                # "System Format"
              }
              frame 2 {
                # "No Used"
                n301 = Equal?(x=w458, y=u16 2) -> (x = y?=w460:bool)
                n302 = Select(t="%x" ("format string"), s=w460, f="") -> (s? t:f=w457:string)
              }
            }
            n303 = Compound Arithmetic op=AND(w422, w421) -> (w414:bool)
            n304 = Compound Arithmetic op=AND(invert w422, w421) -> (w418:bool)
            n305 = Compound Arithmetic op=AND(w422, invert w421) -> (w419:bool)
            n306 = Compound Arithmetic op=AND(invert w422, invert w421) -> (w423:bool)
            n307 = Compound Arithmetic op=OR(w418, w419) -> (w420:bool)
            n308 = Build Array(w414, w420, w423) -> (w415:bool[])
            n309 = Search 1D Array(1D array=w415, element=TRUE) -> (index of element=w417:i32)  [unwired: 1 in]
            n310 = case shown="2" w417 {
              tunnel: [" " ("format string") "" ("format string") "\n" ("format string")] -> w424
              frame 0, Default {
              }
              frame 1 {
              }
              frame 2 {
              }
            }
            n311 = Concatenate Strings("%<" ("string"), w408, w424, w409, ">T" ("string")) -> (w407:string)
          }
        }
        n312 = local read "FormatAxis"() -> (w348:u16)
        n313 = case shown="0, Default" w348 {
          tunnel: w347 -> [w352 w355 w358]
          tunnel: w349 -> [w351 w353 w356]
          frame 0, Default {
            n314 = property class="XYGraph"(reference=w352, "XScale.FormatString"=w351) -> ()  [unwired: 1 in, 2 out]
          }
          frame 1 {
            n315 = property class="XYGraph"(reference=w355, "ActYScl"=0 ("Active Y Scale"), "YScale.FormatString"=w353) -> ()  [unwired: 1 in, 2 out]
          }
          frame 2 {
            n316 = property class="XYGraph"(reference=w358, "ActYScl"=1 ("Active Y Scale"), "YScale.FormatString"=w356) -> ()  [unwired: 1 in, 2 out]
          }
        }
      }
      event "LineStyle0", "LineStyle1", "LineStyle2", "LineStyle3", "LineStyle4": Value Change {
        n317 = event-data() -> ("CtlRef"=w491:refnum<vi>)  [unwired: 6 out]
        n318 = flat-sequence {
          tunnel: w491 -> [w492]
          frame #0 {
            n319 = local write "Plot PropertyCtrl Ref"(w492) -> ()
          }
          frame #1 {
            n320 = property on="Plot Property" class="Str"("Val(Sgnl)"="LineStyle" ("sOption")) -> ()  [unwired: 2 in, 2 out]
          }
        }
      }
      event "LineWidth0", "LineWidth1", "LineWidth2", "LineWidth3", "LineWidth4", "LineWidth5": Value Change {
        n321 = event-data() -> ("CtlRef"=w494:refnum<vi>)  [unwired: 6 out]
        n322 = flat-sequence {
          tunnel: w494 -> [w495]
          frame #0 {
            n323 = local write "Plot PropertyCtrl Ref"(w495) -> ()
          }
          frame #1 {
            n324 = property on="Plot Property" class="Str"("Val(Sgnl)"="LineWidth" ("sOption")) -> ()  [unwired: 2 in, 2 out]
          }
        }
      }
      event "PointStyle0", "PointStyle1", "PointStyle2", "PointStyle3", "PointStyle4", "PointStyle5", "PointStyle6", "PointStyle7", "PointStyle8", "PointStyle9", "PointStyle10", "PointStyle11", "PointStyle12", "PointStyle13", "PointStyle14", "PointStyle15", "PointStyle16": Value Change {
        n325 = event-data() -> ("CtlRef"=w497:refnum<vi>)  [unwired: 6 out]
        n326 = flat-sequence {
          tunnel: w497 -> [w498]
          frame #0 {
            n327 = local write "Plot PropertyCtrl Ref"(w498) -> ()
          }
          frame #1 {
            n328 = property on="Plot Property" class="Str"("Val(Sgnl)"="PointStyle" ("sOption")) -> ()  [unwired: 2 in, 2 out]
          }
        }
      }
      event "Interpolation0", "Interpolation1", "Interpolation2", "Interpolation3", "Interpolation4", "Interpolation5": Value Change {
        n329 = event-data() -> ("CtlRef"=w500:refnum<vi>)  [unwired: 6 out]
        n330 = flat-sequence {
          tunnel: w500 -> [w501]
          frame #0 {
            n331 = local write "Plot PropertyCtrl Ref"(w501) -> ()
          }
          frame #1 {
            n332 = property on="Plot Property" class="Str"("Val(Sgnl)"="Interpolation" ("sOption")) -> ()  [unwired: 2 in, 2 out]
          }
        }
      }
      event "Plot Property": Value Change {
        n333 = event-data() -> ("NewVal"=w503:string)  [unwired: 6 out]
        n334 = case shown="\"LineStyle\", Default" w503 {
          tunnel: [w514 w515 w516 w517] -> w506
          frame "LineStyle", Default {
            n335 = local read "LineStyle"() -> (w514:string)
          }
          frame "LineWidth" {
            n336 = local read "LineWidth"() -> (w515:string)
          }
          frame "PointStyle" {
            n337 = local read "PointStyle"() -> (w516:string)
          }
          frame "Interpolation" {
            n338 = local read "Interpolation"() -> (w517:string)
          }
        }
        n339 = local read "Plot PropertyCtrl Ref"() -> (w505:refnum<vi>)
        n340 = local read "Graph VI Ref"() -> (w508:refnum<vi>)
        n341 = control-ref of="This VI"() -> (w509:refnum<vi>)
        n342 = property on="Items" class="Ring (strict)"() -> ("Value"=w507:u16)  [unwired: 2 in, 2 out]
        n343 = call "CRYChange Plot Property.vi"("Items"=w507, "sOption"=w503, "Control Ref"=w505, "pProperty VI"=w509, "pGraph VI In"=w508, "ControlName In"=w506) -> ("ControlName Out"=w504:string)  [unwired: 5 in]
        n344 = case shown="\"LineStyle\", Default" w503 {
          tunnel: w504 -> [w510 w511 w512 w513]
          frame "LineStyle", Default {
            n345 = local write "LineStyle"(w510) -> ()
          }
          frame "LineWidth" {
            n346 = local write "LineWidth"(w511) -> ()
          }
          frame "PointStyle" {
            n347 = local write "PointStyle"(w512) -> ()
          }
          frame "Interpolation" {
            n348 = local write "Interpolation"(w513) -> ()
          }
        }
      }
      event "Items": Value Change {
        n349 = event-data() -> ("NewVal"=w519:u16)  [unwired: 6 out]
        n350 = flat-sequence {
          tunnel: w518 -> [w528]
          tunnel: w519 -> [w522]
          tunnel: w520 -> [w524]
          tunnel: [w533] -> w521
          tunnel: w521 -> [w542]
          tunnel: w519 -> [w543]
          tunnel: w518 -> [w541]
          frame #0 {
            n351 = property class="MCListbox"(reference=w524) -> ("ItemSyms"=w527:i32[])  [unwired: 1 in, 2 out]
            n352 = Index Array(array=w527, index=w522) -> (element=w525:i32)
            n353 = Equal?(x=w525, y=38) -> (x = y?=w523:bool)
            n354 = property class="XYGraph"(reference=w528, "Active Plot"=w522, "Plot.Visible?"=w523) -> ()  [unwired: 1 in, 2 out]
            n355 = local write "Show Plot"(w523) -> ()
          }
          frame #1 {
            n356 = control-ref of="This VI"() -> (w533:refnum<vi>)
            n357 = local read "Interpolation"() -> (w529:string)
            n358 = local read "LineWidth"() -> (w531:string)
            n359 = local read "PointStyle"() -> (w530:string)
            n360 = local read "LineStyle"() -> (w532:string)
            n361 = To Variant(anything=FALSE) -> (Variant=w535:variant)
            n362 = invoke class="VI" method="Ctrl Val.Set"(reference=w533, "Control Name"=w532, "Value"=w535) -> ()  [unwired: 2 in, 5 out]
            n363 = invoke class="VI" method="Ctrl Val.Set"(reference=w533, "Control Name"=w531, "Value"=w535) -> ()  [unwired: 2 in, 5 out]
            n364 = invoke class="VI" method="Ctrl Val.Set"(reference=w533, "Control Name"=w530, "Value"=w535) -> ()  [unwired: 2 in, 5 out]
            n365 = invoke class="VI" method="Ctrl Val.Set"(reference=w533, "Control Name"=w529, "Value"=w535) -> ()  [unwired: 2 in, 5 out]
          }
          frame #2 {
            n366 = call "CRYGet Line Infor.vi"("This VI"=w542, "Active Plot Number"=w543, "Graph Type"="XY", "XY Graph Control Ref"=w541, "Property Set?"=TRUE) -> ("Line"=w536:u32, "Point/Fill"=w537:u32, "Fill to"=w538:i16, "LineStyle"=w547:string, "LineWidth"=w546:string, "PointStyle"=w545:string, "Interpolation"=w544:string)  [unwired: 16 in]
            n367 = local write "Interpolation"(w544) -> ()
            n368 = local write "LineWidth"(w546) -> ()
            n369 = local write "Point/Fill"(w537) -> ()
            n370 = local write "LineStyle"(w547) -> ()
            n371 = local write "PointStyle"(w545) -> ()
            n372 = local write "Fill to"(w538) -> ()
            n373 = local write "Line"(w536) -> ()
          }
        }
      }
      event "Line": Value Change {
        n374 = event-data() -> ("NewVal"=w553:u32)  [unwired: 6 out]
        n375 = property class="XYGraph"(reference=w555, "Plot.Plot Color"=w553) -> ()  [unwired: 1 in, 2 out]
        n376 = property on="Items" class="Ring (strict)"() -> ("Value"=w550:u16)  [unwired: 2 in, 2 out]
        n377 = Bundle By Name(cluster=T4 {"Row"=0, "Column"=0} ("Active Cell:Active Cell"), "Row"=w550, "Column"=1) -> (w551:T4)
        n378 = property class="MCListbox"(reference=w554, "ActiveCell"=w551, "CellBG"=w553) -> ()  [unwired: 1 in, 2 out]
        n379 = case shown="Default" w548 {
          tunnel: w554 -> [w559 _]
          tunnel: w553 -> [w558 _]
          tunnel: w550 -> [w557 _]
          frame Default {
            n380 = call "CRYSet Plot Settings.vi"("sAction"="Color", "Color"=w558, "Row"=w557, "Legend Refnum"=w559, "Type"=enum16{"Curves", "Values", "Results", "WFM"}."Curves") -> ()  [unwired: 2 in, 5 out]
          }
          frame "ViewReport" {
          }
        }
      }
      event "Point/Fill": Value Change {
        n381 = event-data() -> ("NewVal"=w562:u32)  [unwired: 6 out]
        n382 = property class="XYGraph"(reference=w565, "Plot.Fill/Pt. Color"=w562) -> ()  [unwired: 1 in, 2 out]
        n383 = property on="Items" class="Ring (strict)"() -> ("Value"=w564:u16)  [unwired: 2 in, 2 out]
        n384 = case shown="Default" w563 {
          tunnel: w561 -> [w569 _]
          tunnel: w562 -> [w568 _]
          tunnel: w564 -> [w567 _]
          frame Default {
            n385 = call "CRYSet Plot Settings.vi"("sAction"="PointColor", "Color"=w568, "Row"=w567, "Legend Refnum"=w569, "Type"=enum16{"Curves", "Values", "Results", "WFM"}."Curves") -> ()  [unwired: 2 in, 5 out]
          }
          frame "ViewReport" {
          }
        }
      }
      event "Fill to": Value Change {
        n386 = event-data() -> ("NewVal"=w571:i16)  [unwired: 6 out]
        n387 = property class="XYGraph"(reference=w575, "Plot.Fill To"=w571) -> ()  [unwired: 1 in, 2 out]
        n388 = property on="Items" class="Ring (strict)"() -> ("Value"=w574:u16)  [unwired: 2 in, 2 out]
        n389 = case shown="Default" w572 {
          tunnel: w573 -> [w579 _]
          tunnel: w574 -> [w578 _]
          tunnel: w571 -> [w576 _]
          frame Default {
            n390 = call "CRYSet Plot Settings.vi"("Fill To"=w576, "sAction"="FillTo", "Row"=w578, "Legend Refnum"=w579, "Type"=enum16{"Curves", "Values", "Results", "WFM"}."Curves") -> ()  [unwired: 2 in, 5 out]
          }
          frame "ViewReport" {
          }
        }
      }
      event "Show Plot": Value Change {
        w586 = 38
        n391 = event-data() -> ("NewVal"=w591:bool)  [unwired: 6 out]
        n392 = local read "Items"() -> (w583:u16)
        n393 = property class="MCListbox"(reference=w589) -> (reference out=w588:refnum<vi>, "ItemSyms"=w582:i32[])  [unwired: 1 in, 1 out]
        n394 = property class="XYGraph"(reference=w592, "Active Plot"=w583, "Plot.Visible?"=w591) -> ()  [unwired: 1 in, 2 out]
        n395 = Index Array(array=w582, index=w583) -> (element=w590:i32)
        n396 = Equal?(x=w590, y=w586) -> (x = y?=w587:bool)
        n397 = Select(t=37, s=w587, f=w586) -> (s? t:f=w584:i32)
        n398 = Replace Array Subset(array=w582, new element=w584, index=w583) -> (w581:i32[])
        n399 = property class="MCListbox"(reference=w588, "ItemSyms"=w581) -> ()  [unwired: 1 in, 2 out]
      }
      event "Axis": Value Change {
        n400 = event-data() -> ("NewVal"=w615:u16)  [unwired: 6 out]
        n401 = case shown="1" w615 {
          tunnel: w614 -> [w628 w642 w656]
          tunnel: [w627 w641 w655] -> w613
          tunnel: [w626 w640 w654] -> w610
          tunnel: [w625 w639 w653] -> w608
          tunnel: [w624 w638 w652] -> w605
          tunnel: [w623 w637 w651] -> w604
          tunnel: [w622 w636 w650] -> w603
          tunnel: [w621 w635 w649] -> w602
          tunnel: [w620 w634 w648] -> w601
          tunnel: [w619 w633 w647] -> w600
          tunnel: [w618 w632 w646] -> w599
          tunnel: [w617 w631 w645] -> w598
          tunnel: [w616 w629 w643] -> w597
          frame 0, Default {
            n402 = property class="XYGraph"(reference=w628) -> ("XScale.NameLbl.Visible"=w627:bool, "XScale.Style"=w626:u8, "XScale.Mapping Mode"=w625:u8, "XScale.ScaleFit"=w624:u8, "XScale.Maximum"=w623:dbl, "XScale.Minimum"=w622:dbl, "XScale.TickColor"=w621:u32, "XScale.MinorTickColor"=w620:u32, "XScale.Text Color"=w619:u32, "XScale.MajGrdColor"=w618:u32, "XScale.MnrGrdColor"=w617:u32, "XScale.NameLbl.Text"=w616:string)  [unwired: 1 in, 2 out]
          }
          frame 1 {
            n403 = property class="XYGraph"(reference=w642, "ActYScl"=0 ("Active X Scale")) -> ("YScale.NameLbl.Visible"=w641:bool, "YScale.Style"=w640:u8, "YScale.Mapping Mode"=w639:u8, "YScale.ScaleFit"=w638:u8, "YScale.Maximum"=w637:dbl, "YScale.Minimum"=w636:dbl, "YScale.TickColor"=w635:u32, "YScale.MinorTickColor"=w634:u32, "YScale.Text Color"=w633:u32, "YScale.MajGrdColor"=w632:u32, "YScale.MnrGrdColor"=w631:u32, "YScale.NameLbl.Text"=w629:string)  [unwired: 1 in, 2 out]
          }
          frame 2 {
            n404 = property class="XYGraph"(reference=w656, "ActYScl"=1 ("Active X Scale")) -> ("YScale.NameLbl.Visible"=w655:bool, "YScale.Style"=w654:u8, "YScale.Mapping Mode"=w653:u8, "YScale.ScaleFit"=w652:u8, "YScale.Maximum"=w651:dbl, "YScale.Minimum"=w650:dbl, "YScale.TickColor"=w649:u32, "YScale.MinorTickColor"=w648:u32, "YScale.Text Color"=w647:u32, "YScale.MajGrdColor"=w646:u32, "YScale.MnrGrdColor"=w645:u32, "YScale.NameLbl.Text"=w643:string)  [unwired: 1 in, 2 out]
          }
        }
        n405 = Not Equal?(x=w610, y=u8 5 ("X Scale.Scale Fit")) -> (x != y?=w611:bool)
        n406 = Equal?(x=w608, y=u8 1 ("X Scale.Scale Fit")) -> (x = y?=w607:bool)
        n407 = Equal?(x=w605, y=u8 2 ("X Scale.Scale Fit")) -> (x = y?=w593:bool)
        n408 = local write "Show scale label"(w613) -> ()
        n409 = local write "Minor grid"(w598) -> ()
        n410 = local write "Minimum"(w603) -> ()
        n411 = local write "Minor tick"(w601) -> ()
        n412 = local write "Major grid"(w599) -> ()
        n413 = local write "Axis Name"(w597) -> ()
        n414 = local write "Show scale"(w611) -> ()
        n415 = local write "Maximum"(w604) -> ()
        n416 = local write "Major tick"(w602) -> ()
        n417 = local write "Marker text"(w600) -> ()
        n418 = local write "Autoscale"(w593) -> ()
        n419 = local write "Scale Style"(w610) -> ()
        n420 = local write "Log"(w607) -> ()
        n421 = Select(t=u8 2 ("X Scale.Scale Fit"), s=w593, f=u8 0 ("X Scale.Scale Fit")) -> (s? t:f=w594:u8)
        n422 = property on="Maximum" class="DigNum (strict)"("Disabled"=w594) -> ()  [unwired: 2 in, 2 out]
        n423 = property on="Minimum" class="DigNum (strict)"("Disabled"=w594) -> ()  [unwired: 2 in, 2 out]
      }
      event "Axis Name": Value Change {
        n424 = event-data() -> ("NewVal"=w657:string)  [unwired: 6 out]
        n425 = local write "Axis Name"(w657) -> ()
        n426 = local read "Axis"() -> (w659:u16)
        n427 = case shown="2" w659 {
          tunnel: w658 -> [w661 w664 w667]
          tunnel: w657 -> [w660 w662 w665]
          frame 0, Default {
            n428 = property class="XYGraph"(reference=w661, "XScale.NameLbl.Text"=w660) -> ()  [unwired: 1 in, 2 out]
          }
          frame 1 {
            n429 = property class="XYGraph"(reference=w664, "ActYScl"=0 ("Active Y Scale"), "YScale.NameLbl.Text"=w662) -> ()  [unwired: 1 in, 2 out]
          }
          frame 2 {
            n430 = property class="XYGraph"(reference=w667, "ActYScl"=1 ("Active Y Scale"), "YScale.NameLbl.Text"=w665) -> ()  [unwired: 1 in, 2 out]
          }
        }
      }
      event "Show scale label": Value Change {
        n431 = event-data() -> ("NewVal"=w668:bool)  [unwired: 6 out]
        n432 = local read "Axis"() -> (w669:u16)
        n433 = case shown="2" w669 {
          tunnel: w670 -> [w672 w675 w678]
          tunnel: w668 -> [w671 w673 w676]
          frame 0, Default {
            n434 = property class="XYGraph"(reference=w672, "XScale.NameLbl.Visible"=w671) -> ()  [unwired: 1 in, 2 out]
          }
          frame 1 {
            n435 = property class="XYGraph"(reference=w675, "ActYScl"=0 ("Active Y Scale"), "YScale.NameLbl.Visible"=w673) -> ()  [unwired: 1 in, 2 out]
          }
          frame 2 {
            n436 = property class="XYGraph"(reference=w678, "ActYScl"=1 ("Active Y Scale"), "YScale.NameLbl.Visible"=w676) -> ()  [unwired: 1 in, 2 out]
          }
        }
      }
      event "Show scale": Value Change {
        n437 = event-data() -> ("NewVal"=w687:bool)  [unwired: 6 out]
        n438 = local read "Scale Style"() -> (w680:u8)
        n439 = Equal?(x=u8 5 ("X Scale.Scale Fit"), y=w680) -> (x = y?=w682:bool)
        n440 = Select(t=u8 0 ("X Scale.Scale Fit"), s=w682, f=w680) -> (s? t:f=w679:u8)
        n441 = Select(t=w679, s=w687, f=u8 5 ("X Scale.Scale Fit")) -> (s? t:f=w684:u8)
        n442 = local write "Scale Style"(w684) -> ()
        n443 = local read "Axis"() -> (w686:u16)
        n444 = case shown="1" w686 {
          tunnel: w684 -> [w690 w692 w694]
          tunnel: w685 -> [w689 w693 w696]
          frame 0, Default {
            n445 = property class="XYGraph"(reference=w689, "XScale.Style"=w690) -> ()  [unwired: 1 in, 2 out]
          }
          frame 1 {
            n446 = property class="XYGraph"(reference=w693, "ActYScl"=0 ("Active Y Scale"), "YScale.Style"=w692) -> ()  [unwired: 1 in, 2 out]
          }
          frame 2 {
            n447 = property class="XYGraph"(reference=w696, "ActYScl"=1 ("Active Y Scale"), "YScale.Style"=w694) -> ()  [unwired: 1 in, 2 out]
          }
        }
      }
      event "Log": Value Change {
        n448 = event-data() -> ("NewVal"=w700:bool)  [unwired: 6 out]
        n449 = Select(t=u8 1 ("X Scale.Scale Fit"), s=w700, f=u8 0 ("X Scale.Scale Fit")) -> (s? t:f=w698:u8)
        n450 = local read "Axis"() -> (w699:u16)
        n451 = case shown="2" w699 {
          tunnel: w698 -> [w704 w706 w708]
          tunnel: w697 -> [w703 w707 w710]
          frame 0, Default {
            n452 = property class="XYGraph"(reference=w703, "XScale.Mapping Mode"=w704) -> ()  [unwired: 1 in, 2 out]
          }
          frame 1 {
            n453 = property class="XYGraph"(reference=w707, "ActYScl"=0 ("Active Y Scale"), "YScale.Mapping Mode"=w706) -> ()  [unwired: 1 in, 2 out]
          }
          frame 2 {
            n454 = property class="XYGraph"(reference=w710, "ActYScl"=1 ("Active Y Scale"), "YScale.Mapping Mode"=w708) -> ()  [unwired: 1 in, 2 out]
          }
        }
      }
      event "GridStyle": Value Change {
        n455 = event-data() -> ("NewVal"=w712:u16)  [unwired: 6 out]
        n456 = local read "Axis"() -> (w713:u16)
        n457 = case shown="2" w713 {
          tunnel: w712 -> [w715 w717 w719]
          tunnel: w711 -> [w714 w718 w721]
          frame 0, Default {
            n458 = property class="XYGraph"(reference=w714, "XScale.Style"=w715) -> ()  [unwired: 1 in, 2 out]
          }
          frame 1 {
            n459 = property class="XYGraph"(reference=w718, "ActYScl"=0 ("Active Y Scale"), "YScale.Style"=w717) -> ()  [unwired: 1 in, 2 out]
          }
          frame 2 {
            n460 = property class="XYGraph"(reference=w721, "ActYScl"=1 ("Active Y Scale"), "YScale.Style"=w719) -> ()  [unwired: 1 in, 2 out]
          }
        }
      }
      event "Major tick": Value Change {
        n461 = event-data() -> ("NewVal"=w722:u32)  [unwired: 6 out]
        n462 = local read "Axis"() -> (w724:u16)
        n463 = case shown="0, Default" w724 {
          tunnel: w723 -> [w726 w729 w732]
          tunnel: w722 -> [w725 w727 w730]
          frame 0, Default {
            n464 = property class="XYGraph"(reference=w726, "XScale.TickColor"=w725) -> ()  [unwired: 1 in, 2 out]
          }
          frame 1 {
            n465 = property class="XYGraph"(reference=w729, "ActYScl"=0 ("Active Y Scale"), "YScale.TickColor"=w727) -> ()  [unwired: 1 in, 2 out]
          }
          frame 2 {
            n466 = property class="XYGraph"(reference=w732, "ActYScl"=1 ("Active Y Scale"), "YScale.TickColor"=w730) -> ()  [unwired: 1 in, 2 out]
          }
        }
      }
      event "Minor tick": Value Change {
        n467 = event-data() -> ("NewVal"=w733:u32)  [unwired: 6 out]
        n468 = local read "Axis"() -> (w735:u16)
        n469 = case shown="0, Default" w735 {
          tunnel: w733 -> [w737 w739 w741]
          tunnel: w734 -> [w736 w740 w743]
          frame 0, Default {
            n470 = property class="XYGraph"(reference=w736, "XScale.MinorTickColor"=w737) -> ()  [unwired: 1 in, 2 out]
          }
          frame 1 {
            n471 = property class="XYGraph"(reference=w740, "ActYScl"=0 ("Active Y Scale"), "YScale.MinorTickColor"=w739) -> ()  [unwired: 1 in, 2 out]
          }
          frame 2 {
            n472 = property class="XYGraph"(reference=w743, "ActYScl"=1 ("Active Y Scale"), "YScale.MinorTickColor"=w741) -> ()  [unwired: 1 in, 2 out]
          }
        }
      }
      event "Marker text": Value Change {
        n473 = event-data() -> ("NewVal"=w744:u32)  [unwired: 6 out]
        n474 = local read "Axis"() -> (w746:u16)
        n475 = case shown="0, Default" w746 {
          tunnel: w744 -> [w748 w750 w752]
          tunnel: w745 -> [w747 w751 w754]
          frame 0, Default {
            n476 = property class="XYGraph"(reference=w747, "XScale.Text Color"=w748) -> ()  [unwired: 1 in, 2 out]
          }
          frame 1 {
            n477 = property class="XYGraph"(reference=w751, "ActYScl"=0 ("Active Y Scale"), "YScale.Text Color"=w750) -> ()  [unwired: 1 in, 2 out]
          }
          frame 2 {
            n478 = property class="XYGraph"(reference=w754, "ActYScl"=1 ("Active Y Scale"), "YScale.Text Color"=w752) -> ()  [unwired: 1 in, 2 out]
          }
        }
      }
      event "Major grid": Value Change {
        n479 = event-data() -> ("NewVal"=w756:u32)  [unwired: 6 out]
        n480 = local read "Axis"() -> (w757:u16)
        n481 = case shown="0, Default" w757 {
          tunnel: w756 -> [w759 w761 w763]
          tunnel: w755 -> [w758 w762 w765]
          frame 0, Default {
            n482 = property class="XYGraph"(reference=w758, "XScale.MajGrdColor"=w759) -> ()  [unwired: 1 in, 2 out]
          }
          frame 1 {
            n483 = property class="XYGraph"(reference=w762, "ActYScl"=0 ("Active Y Scale"), "YScale.MajGrdColor"=w761) -> ()  [unwired: 1 in, 2 out]
          }
          frame 2 {
            n484 = property class="XYGraph"(reference=w765, "ActYScl"=1 ("Active Y Scale"), "YScale.MajGrdColor"=w763) -> ()  [unwired: 1 in, 2 out]
          }
        }
      }
      event "Minor grid": Value Change {
        n485 = event-data() -> ("NewVal"=w766:u32)  [unwired: 6 out]
        n486 = local read "Axis"() -> (w768:u16)
        n487 = case shown="0, Default" w768 {
          tunnel: w766 -> [w770 w772 w774]
          tunnel: w767 -> [w769 w773 w776]
          frame 0, Default {
            n488 = property class="XYGraph"(reference=w769, "XScale.MnrGrdColor"=w770) -> ()  [unwired: 1 in, 2 out]
          }
          frame 1 {
            n489 = property class="XYGraph"(reference=w773, "ActYScl"=0 ("Active Y Scale"), "YScale.MnrGrdColor"=w772) -> ()  [unwired: 1 in, 2 out]
          }
          frame 2 {
            n490 = property class="XYGraph"(reference=w776, "ActYScl"=1 ("Active Y Scale"), "YScale.MnrGrdColor"=w774) -> ()  [unwired: 1 in, 2 out]
          }
        }
      }
      event "Autoscale": Value Change {
        n491 = event-data() -> ("NewVal"=w778:bool)  [unwired: 6 out]
        n492 = local read "Axis"() -> (w788:u16)
        n493 = Select(t=u8 2 ("X Scale.Scale Fit"), s=w778, f=u8 0 ("X Scale.Scale Fit")) -> (s? t:f=w792:u8)
        n494 = local read "Maximum"() -> (w787:dbl)
        n495 = local read "Minimum"() -> (w786:dbl)
        n496 = Select(t=u8 2 ("X Scale.Scale Fit"), s=w778, f=u8 0 ("X Scale.Scale Fit")) -> (s? t:f=w791:u8)
        n497 = case shown="False" w778 {
          tunnel: w788 -> [w798 _]
          tunnel: w787 -> [w797 _]
          tunnel: w786 -> [w796 _]
          tunnel: w785 -> [w795 _]
          frame False {
            n498 = case shown="0, Default" w798 {
              tunnel: w795 -> [w801 w805 w809]
              tunnel: w797 -> [w800 w803 w807]
              tunnel: w796 -> [w799 w802 w806]
              frame 0, Default {
                n499 = property class="XYGraph"(reference=w801, "XScale.Maximum"=w800, "XScale.Minimum"=w799) -> ()  [unwired: 1 in, 2 out]
              }
              frame 1 {
                n500 = property class="XYGraph"(reference=w805, "ActYScl"=0 ("Active Y Scale"), "YScale.Maximum"=w803, "YScale.Minimum"=w802) -> ()  [unwired: 1 in, 2 out]
              }
              frame 2 {
                n501 = property class="XYGraph"(reference=w809, "ActYScl"=1 ("Active Y Scale"), "YScale.Maximum"=w807, "YScale.Minimum"=w806) -> ()  [unwired: 1 in, 2 out]
              }
            }
          }
          frame True {
          }
        }
        n502 = case shown="2" w788 {
          tunnel: w792 -> [w811 w815 w818]
          tunnel: w785 -> [w812 w816 w820]
          tunnel: ["ScaleFitX" ("Label Name") "ScaleFitY" ("Label Name") "ScaleFitY 2" ("Label Name")] -> w783
          frame 0, Default {
            n503 = property class="XYGraph"(reference=w812, "XScale.ScaleFit"=w811) -> ()  [unwired: 1 in, 2 out]
          }
          frame 1 {
            n504 = property class="XYGraph"(reference=w816, "ActYScl"=0 ("Active Y Scale"), "YScale.ScaleFit"=w815) -> ()  [unwired: 1 in, 2 out]
          }
          frame 2 {
            n505 = property class="XYGraph"(reference=w820, "ActYScl"=1 ("Active Y Scale"), "YScale.ScaleFit"=w818) -> ()  [unwired: 1 in, 2 out]
          }
        }
        n506 = property on="Maximum" class="DigNum (strict)"("Disabled"=w791) -> ()  [unwired: 2 in, 2 out]
        n507 = property on="Minimum" class="DigNum (strict)"("Disabled"=w791) -> ()  [unwired: 2 in, 2 out]
        n508 = call "CRYGet Boolean Reference.vi"("Label Name"=w783, "VI Refnum"=w784) -> ("Boolean Ref"=w782:refnum<vi>, "VI Refnum Out"=w781:refnum<vi>)  [unwired: 7 in, 1 out]
        n509 = property class="Bool"(reference=w782, "Value"=w778) -> (error out=w777:errorcluster)  [unwired: 1 in, 1 out]
        n510 = call "CRYGet Boolean Reference.vi"("Label Name"="ToolbarUpdate", "VI Refnum"=w781) -> ("Boolean Ref"=w779:refnum<vi>)  [unwired: 7 in, 2 out]
        n511 = property class="Bool"(reference=w779, error in=w777, "Val(Sgnl)"=w778) -> ()  [unwired: 2 out]
      }
      event "Maximum": Value Change {
        n512 = event-data() -> ("NewVal"=w821:dbl)  [unwired: 6 out]
        n513 = local read "Axis"() -> (w823:u16)
        n514 = case shown="0, Default" w823 {
          tunnel: w821 -> [w825 w827 w829]
          tunnel: w822 -> [w824 w828 w831]
          frame 0, Default {
            n515 = property class="XYGraph"(reference=w824, "XScale.Maximum"=w825) -> ()  [unwired: 1 in, 2 out]
          }
          frame 1 {
            n516 = property class="XYGraph"(reference=w828, "ActYScl"=0 ("Active Y Scale"), "YScale.Maximum"=w827) -> ()  [unwired: 1 in, 2 out]
          }
          frame 2 {
            n517 = property class="XYGraph"(reference=w831, "ActYScl"=1 ("Active Y Scale"), "YScale.Maximum"=w829) -> ()  [unwired: 1 in, 2 out]
          }
        }
        n518 = local write "Maximum"(w821) -> ()
      }
      event "Minimum": Value Change {
        n519 = event-data() -> ("NewVal"=w832:dbl)  [unwired: 6 out]
        n520 = local read "Axis"() -> (w834:u16)
        n521 = case shown="0, Default" w834 {
          tunnel: w832 -> [w836 w838 w840]
          tunnel: w833 -> [w835 w839 w842]
          frame 0, Default {
            n522 = property class="XYGraph"(reference=w835, "XScale.Minimum"=w836) -> ()  [unwired: 1 in, 2 out]
          }
          frame 1 {
            n523 = property class="XYGraph"(reference=w839, "ActYScl"=0 ("Active Y Scale"), "YScale.Minimum"=w838) -> ()  [unwired: 1 in, 2 out]
          }
          frame 2 {
            n524 = property class="XYGraph"(reference=w842, "ActYScl"=1 ("Active Y Scale"), "YScale.Minimum"=w840) -> ()  [unwired: 1 in, 2 out]
          }
        }
        n525 = local write "Minimum"(w832) -> ()
      }
      event "Show Cursors": Value Change {
        n526 = event-data() -> ("NewVal"=w843:bool)  [unwired: 6 out]
        n527 = local write "Show Cursors"(w843) -> ()
        n528 = Select(t=0, s=w843, f=2) -> (s? t:f=w847:i32)
        n529 = call "CRYGet Boolean Reference.vi"("Label Name"="CursorShow", "VI Refnum"=w846) -> ("Boolean Ref"=w845:refnum<vi>)  [unwired: 7 in, 2 out]
        n530 = property on="Cursor Tab" class="TabCtl (strict)"("DisabledEnum"=w847) -> ()  [unwired: 2 in, 2 out]
        n531 = property class="Bool"(reference=w845, "Val(Sgnl)"=w843) -> ()  [unwired: 1 in, 2 out]
      }
      event "Cursor Items": Value Change {
        n532 = event-data() -> ("NewVal"=w851:u16)  [unwired: 6 out]
        n533 = flat-sequence {
          tunnel: [w858] -> w852
          tunnel: w852 -> [w862]
          tunnel: w851 -> [w860]
          tunnel: w850 -> [w861]
          frame #0 {
            n534 = local read "CursorLineWidth"() -> (w856:string)
            n535 = local read "CursorPointStyle"() -> (w855:string)
            n536 = local read "CursorLineStyle"() -> (w857:string)
            n537 = control-ref of="This VI"() -> (w858:refnum<vi>)
            n538 = local read "CursorStyle"() -> (w854:string)
            n539 = To Variant(anything=FALSE) -> (Variant=w859:variant)
            n540 = invoke class="VI" method="Ctrl Val.Set"(reference=w858, "Control Name"=w857, "Value"=w859) -> ()  [unwired: 2 in, 5 out]
            n541 = invoke class="VI" method="Ctrl Val.Set"(reference=w858, "Control Name"=w856, "Value"=w859) -> ()  [unwired: 2 in, 5 out]
            n542 = invoke class="VI" method="Ctrl Val.Set"(reference=w858, "Control Name"=w855, "Value"=w859) -> ()  [unwired: 2 in, 5 out]
            n543 = invoke class="VI" method="Ctrl Val.Set"(reference=w858, "Control Name"=w854, "Value"=w859) -> ()  [unwired: 2 in, 5 out]
          }
          frame #1 {
            n544 = call "CRYSet Cursor Infor.vi"("This VI"=w862, "Active Cursor"=w860, "Graph Type"="XY", "XY Graph Ref"=w861, "Property Set?"=TRUE) -> ("Cursor Color"=w863:u32, "CursorLineStyle"=w866:string, "CursorLineWidth"=w867:string, "CursorPointStyle"=w868:string, "CursorStyle"=w869:string)  [unwired: 17 in, 1 out]
            n545 = local write "CursorLineWidth"(w867) -> ()
            n546 = local write "Cursor color"(w863) -> ()
            n547 = local write "CursorLineStyle"(w866) -> ()
            n548 = local write "CursorPointStyle"(w868) -> ()
            n549 = local write "CursorStyle"(w869) -> ()
          }
        }
      }
      event "CursorLineStyle0", "CursorLineStyle1", "CursorLineStyle2", "CursorLineStyle3", "CursorLineStyle4": Value Change {
        n550 = event-data() -> ("CtlRef"=w871:refnum<vi>)  [unwired: 6 out]
        n551 = local read "CursorLineStyle"() -> (w872:string)
        n552 = property class="Bool (strict)"(reference=w871) -> ("Label.Text"=w873:string)  [unwired: 1 in, 2 out]
        n553 = Equal?(x=w873, y=w872) -> (x = y?=w874:bool)
        n554 = case shown="False" w874 {
          tunnel: w873 -> [w879 w887]
          tunnel: w872 -> [w885 _]
          tunnel: w870 -> [w875 _]
          frame False {
            n555 = control-ref of="This VI"() -> (w886:refnum<vi>)
            n556 = Match Pattern(string=w879, regular expression="CursorLineStyle") -> (after substring=w877:string)  [unwired: 4 out]
            n557 = To Variant(anything=TRUE) -> (Variant=w883:variant)
            n558 = Decimal String To Number(string=w877) -> (number=w876:i32)  [unwired: 3 out]
            n559 = invoke class="VI" method="Ctrl Val.Set"(reference=w886, "Control Name"=w879, "Value"=w883) -> (reference out=w884:refnum<vi>)  [unwired: 2 in, 4 out]
            n560 = local write "CursorLineStyle"(w879) -> ()
            n561 = property class="XYGraph"(reference=w875, "Cursor.LineStyle"=w876) -> ()  [unwired: 1 in, 2 out]
            n562 = To Variant(anything=FALSE) -> (Variant=w881:variant)
            n563 = invoke class="VI" method="Ctrl Val.Set"(reference=w884, "Control Name"=w885, "Value"=w881) -> ()  [unwired: 2 in, 5 out]
          }
          frame True {
            n564 = control-ref of="This VI"() -> (w890:refnum<vi>)
            n565 = To Variant(anything=TRUE) -> (Variant=w889:variant)
            n566 = invoke class="VI" method="Ctrl Val.Set"(reference=w890, "Control Name"=w887, "Value"=w889) -> ()  [unwired: 2 in, 5 out]
          }
        }
      }
      event "CursorLineWidth0", "CursorLineWidth1", "CursorLineWidth2", "CursorLineWidth3", "CursorLineWidth4", "CursorLineWidth5": Value Change {
        n567 = event-data() -> ("CtlRef"=w892:refnum<vi>)  [unwired: 6 out]
        n568 = local read "CursorLineWidth"() -> (w893:string)
        n569 = property class="Bool (strict)"(reference=w892) -> ("Label.Text"=w894:string)  [unwired: 1 in, 2 out]
        n570 = Equal?(x=w894, y=w893) -> (x = y?=w895:bool)
        n571 = case shown="False" w895 {
          tunnel: w894 -> [w898 w908]
          tunnel: w893 -> [w906 _]
          tunnel: w891 -> [w896 _]
          frame False {
            n572 = control-ref of="This VI"() -> (w907:refnum<vi>)
            n573 = Match Pattern(string=w898, regular expression="CursorLineWidth") -> (after substring=w899:string)  [unwired: 4 out]
            n574 = To Variant(anything=TRUE) -> (Variant=w904:variant)
            n575 = Decimal String To Number(string=w899) -> (number=w900:i32)  [unwired: 3 out]
            n576 = invoke class="VI" method="Ctrl Val.Set"(reference=w907, "Control Name"=w898, "Value"=w904) -> (reference out=w905:refnum<vi>)  [unwired: 2 in, 4 out]
            n577 = local write "CursorLineWidth"(w898) -> ()
            n578 = property class="XYGraph"(reference=w896, "Cursor.LineWidth"=w900) -> ()  [unwired: 1 in, 2 out]
            n579 = To Variant(anything=FALSE) -> (Variant=w902:variant)
            n580 = invoke class="VI" method="Ctrl Val.Set"(reference=w905, "Control Name"=w906, "Value"=w902) -> ()  [unwired: 2 in, 5 out]
          }
          frame True {
            n581 = control-ref of="This VI"() -> (w911:refnum<vi>)
            n582 = To Variant(anything=TRUE) -> (Variant=w910:variant)
            n583 = invoke class="VI" method="Ctrl Val.Set"(reference=w911, "Control Name"=w908, "Value"=w910) -> ()  [unwired: 2 in, 5 out]
          }
        }
      }
      event "CursorPointStyle0", "CursorPointStyle1", "CursorPointStyle2", "CursorPointStyle3", "CursorPointStyle4", "CursorPointStyle5", "CursorPointStyle6", "CursorPointStyle7", "CursorPointStyle8", "CursorPointStyle9", "CursorPointStyle10", "CursorPointStyle11", "CursorPointStyle12", "CursorPointStyle13", "CursorPointStyle14", "CursorPointStyle15", "CursorPointStyle16": Value Change {
        n584 = event-data() -> ("CtlRef"=w913:refnum<vi>)  [unwired: 6 out]
        n585 = local read "CursorPointStyle"() -> (w914:string)
        n586 = property class="Bool (strict)"(reference=w913) -> ("Label.Text"=w915:string)  [unwired: 1 in, 2 out]
        n587 = Equal?(x=w915, y=w914) -> (x = y?=w916:bool)
        n588 = case shown="False" w916 {
          tunnel: w915 -> [w919 w929]
          tunnel: w914 -> [w927 _]
          tunnel: w912 -> [w917 _]
          frame False {
            n589 = control-ref of="This VI"() -> (w928:refnum<vi>)
            n590 = To Variant(anything=TRUE) -> (Variant=w925:variant)
            n591 = Match Pattern(string=w919, regular expression="CursorPointStyle") -> (after substring=w920:string)  [unwired: 4 out]
            n592 = invoke class="VI" method="Ctrl Val.Set"(reference=w928, "Control Name"=w919, "Value"=w925) -> (reference out=w926:refnum<vi>)  [unwired: 2 in, 4 out]
            n593 = local write "CursorPointStyle"(w919) -> ()
            n594 = Decimal String To Number(string=w920) -> (number=w921:i32)  [unwired: 3 out]
            n595 = property class="XYGraph"(reference=w917, "Cursor.Cursor Point Style"=w921) -> ()  [unwired: 1 in, 2 out]
            n596 = To Variant(anything=FALSE) -> (Variant=w923:variant)
            n597 = invoke class="VI" method="Ctrl Val.Set"(reference=w926, "Control Name"=w927, "Value"=w923) -> ()  [unwired: 2 in, 5 out]
          }
          frame True {
            n598 = control-ref of="This VI"() -> (w932:refnum<vi>)
            n599 = To Variant(anything=TRUE) -> (Variant=w931:variant)
            n600 = invoke class="VI" method="Ctrl Val.Set"(reference=w932, "Control Name"=w929, "Value"=w931) -> ()  [unwired: 2 in, 5 out]
          }
        }
      }
      event "CursorStyle0", "CursorStyle1", "CursorStyle2", "CursorStyle3", "CursorStyle6", "CursorStyle7", "CursorStyle5", "CursorStyle4", "CursorStyle8": Value Change {
        n601 = event-data() -> ("CtlRef"=w934:refnum<vi>)  [unwired: 6 out]
        n602 = local read "CursorStyle"() -> (w935:string)
        n603 = property class="Bool (strict)"(reference=w934) -> ("Label.Text"=w936:string)  [unwired: 1 in, 2 out]
        n604 = Equal?(x=w936, y=w935) -> (x = y?=w937:bool)
        n605 = case shown="False" w937 {
          tunnel: w936 -> [w940 w950]
          tunnel: w935 -> [w948 _]
          tunnel: w933 -> [w938 _]
          frame False {
            n606 = control-ref of="This VI"() -> (w949:refnum<vi>)
            n607 = To Variant(anything=TRUE) -> (Variant=w946:variant)
            n608 = Match Pattern(string=w940, regular expression="CursorStyle") -> (after substring=w941:string)  [unwired: 4 out]
            n609 = invoke class="VI" method="Ctrl Val.Set"(reference=w949, "Control Name"=w940, "Value"=w946) -> (reference out=w947:refnum<vi>)  [unwired: 2 in, 4 out]
            n610 = Decimal String To Number(string=w941) -> (number=w942:i32)  [unwired: 3 out]
            n611 = local write "CursorStyle"(w940) -> ()
            n612 = property class="XYGraph"(reference=w938, "Cursor.Cursor Style"=w942) -> ()  [unwired: 1 in, 2 out]
            n613 = To Variant(anything=FALSE) -> (Variant=w944:variant)
            n614 = invoke class="VI" method="Ctrl Val.Set"(reference=w947, "Control Name"=w948, "Value"=w944) -> ()  [unwired: 2 in, 5 out]
          }
          frame True {
            n615 = control-ref of="This VI"() -> (w953:refnum<vi>)
            n616 = To Variant(anything=TRUE) -> (Variant=w952:variant)
            n617 = invoke class="VI" method="Ctrl Val.Set"(reference=w953, "Control Name"=w950, "Value"=w952) -> ()  [unwired: 2 in, 5 out]
          }
        }
      }
      event "Cursor color": Value Change {
        n618 = event-data() -> ("NewVal"=w961:u32)  [unwired: 6 out]
        n619 = local read "Cursor Items"() -> (w960:u16)
        n620 = property class="XYGraph"(reference=w958) -> (reference out=w957:refnum<vi>, "Active Cursor"=w955:u32)  [unwired: 1 in, 1 out]
        n621 = local write "Cursor color"(w961) -> ()
        n622 = property class="XYGraph"(reference=w957, "Active Cursor"=w960, "Cursor.Cursor Color"=w961) -> (reference out=w956:refnum<vi>)  [unwired: 1 in, 1 out]
        n623 = property class="XYGraph"(reference=w956, "Active Cursor"=w955) -> (reference out=w954:refnum<vi>)  [unwired: 1 in, 1 out]
        n624 = flat-sequence {
          tunnel: w959 -> [w962]
          tunnel: w954 -> [_]
          frame #0 {
            n625 = call "CRYGet Boolean Reference.vi"("Label Name"="CursorColor" ("Control Name"), "VI Refnum"=w962) -> ("Boolean Ref"=w964:refnum<vi>)  [unwired: 7 in, 2 out]
            n626 = property class="Bool"(reference=w964, "Val(Sgnl)"=TRUE ("Visible")) -> ()  [unwired: 1 in, 2 out]
          }
        }
      }
      event "Linked to plot:": Value Change {
        n627 = event-data() -> ("NewVal"=w977:u16)  [unwired: 6 out]
        n628 = local write "Linked to plot:"(w977) -> ()
        n629 = local read "Cursor Items"() -> (w967:u16)
        n630 = property class="XYGraph"(reference=w978, "Active Cursor"=w967, "Cursor.Cursor Plot"=w977) -> (reference out=w968:refnum<vi>)  [unwired: 1 in, 1 out]
        n631 = property class="Tbl"(reference=w976) -> ("Value"=w975:string[][])  [unwired: 1 in, 2 out]
        n632 = Index Array(array=w975, index (row)=w967) -> (element=w974:string[])  [unwired: 1 in]
        n633 = Index Array(array=w974, index=1) -> (element=w972:string)
        n634 = Match Pattern(string=w972, regular expression=":" ("string")) -> (after substring=w969:string, offset past match=w970:i32)  [unwired: 1 in, 2 out]
        n635 = case shown="1.." w970 {
          tunnel: w969 -> [w984 _]
          tunnel: w968 -> [w982 _]
          tunnel: w967 -> [w981 _]
          tunnel: w966 -> [w979 _]
          frame 1.. {
            n636 = Fract/Exp String To Number(string=w984) -> (number=w983:dbl)  [unwired: 3 in, 1 out]
            n637 = property class="XYGraph"(reference=w982, "Active Cursor"=w981, "Cursor.Cursor X"=w983) -> (reference out=w980:refnum<vi>)  [unwired: 1 in, 1 out]
            n638 = flat-sequence {
              tunnel: w980 -> [_]
              tunnel: w979 -> [w987]
              frame #0 {
                n639 = call "CRYGet Boolean Reference.vi"("Label Name"="CursorPlot", "VI Refnum"=w987) -> ("Boolean Ref"=w986:refnum<vi>)  [unwired: 7 in, 2 out]
                n640 = property class="Bool"(reference=w986, "Val(Sgnl)"=TRUE) -> ()  [unwired: 1 in, 2 out]
              }
            }
          }
          frame ..0 {
          }
        }
      }
      event "Link Cursors": Value Change {
        n641 = event-data() -> ("NewVal"=w989:bool)  [unwired: 6 out]
        n642 = local write "Link Cursors"(w989) -> ()
      }
    }
  }
